vi "Preset_Manager_Main.vi"(4 "Virtual Devices List":string[](array[string]), 6 "Filtered Devices List":string[](array[string]), 8 "Experiment Name":string, 10 "DevStatusQueue":refnum<queue>, 11 "Software Root":string) -> ()   [LabVIEW 2020]
uses:
  <vilib>/Utility/miscctls.llb/LVRowAndColumnTypeDef.ctl
  Preset Query Enum.ctl
  <vilib>/Platform/browser.llb/Open URL in Default Browser (string).vi
  <userlib>/_OpenG.lib/array/array.llb/Delete Elements from 1D Array (String)__ogtk.vi
  <userlib>/_OpenG.lib/array/array.llb/Empty 1D Array (String)__ogtk.vi
panel:
  out "Queue Progress Bar":ext(slide) scale=0.0..1.0
  out "Queue Size":i32
  out "Current Preset Queue Element":string
  in  "Expt Devices Not On":i32(listbox)
  in  "Preset Devices Not in Experiment":i32(listbox)
  out "Active Preset":string
  out "Preset Execution Indicator":bool
  in  "EXIT":bool
  in  "Using Queue":bool
  in  "Tab Control":T1(tab)
  in  "Execute Preset":bool
  in  "Delete Preset":bool
  in  "Save as Preset":bool
  in  "Preset Menu":u16(ring) items=["None", "Pulsed Alignment", "3J", "Diode", "26J", "SingleShot", "1Hz", "800 MAX ND", "Amp3-8J-CapExit", "SDI", "CapInHexPosition", "CapOutHexFiberPosition", "Full Heater, Frog Out", "Full Heater, Frog In", "MagSpecSimulateBoff", "Pulsed", "CW", "Amp2, Clunker In", "Amp3-17J", "MagSpecSimulateBon", "SMFiber-In", "SMFiber-Out", "Amp3-MegaAttenuator", "developer", "developer_main", "developer_test_1", "dev_simcam_2", "dev_simcam_3"]
  in  "Load ECS to Table":bool
  in  "Navigate to ECS File":path
  in  "Preset Table Control":string[][](table)
  in  "Choose Values":bool
  in  "Left Join":bool
  in  "Reset Queue":bool
  in  "Queue Table Control":string[][](table)
  in  "Queue Table":string[][](table)
  in  "Execute Queue":bool
  in  "HELP WEB PAGE":bool
  out "PRESET FROM DB":string[][](table)
  out "ECS File":string[][](table)
  out "Coordinate Array":i32[][](array[numeric])
  out "Devices not started":string[](array[string]) caption="Devices not ready for scan"
  out "Active Device array":bool[](array[boolean])
  out "Active Dev/IP":string[](array[string])
  out "Device Errors":string[][](array[string])
  out "Queue Element":i32
  in  "Poll Count":i32
  in  "Mcast address":string
  in  "MCast Remote":u16
  in  "UDP timeout ms":i32
  in  "MC Multicast":refnum<k16>
  in  "My IP":string
  in  "All Devices Core Info":string[][](array[string])
  out "error out":errorcluster
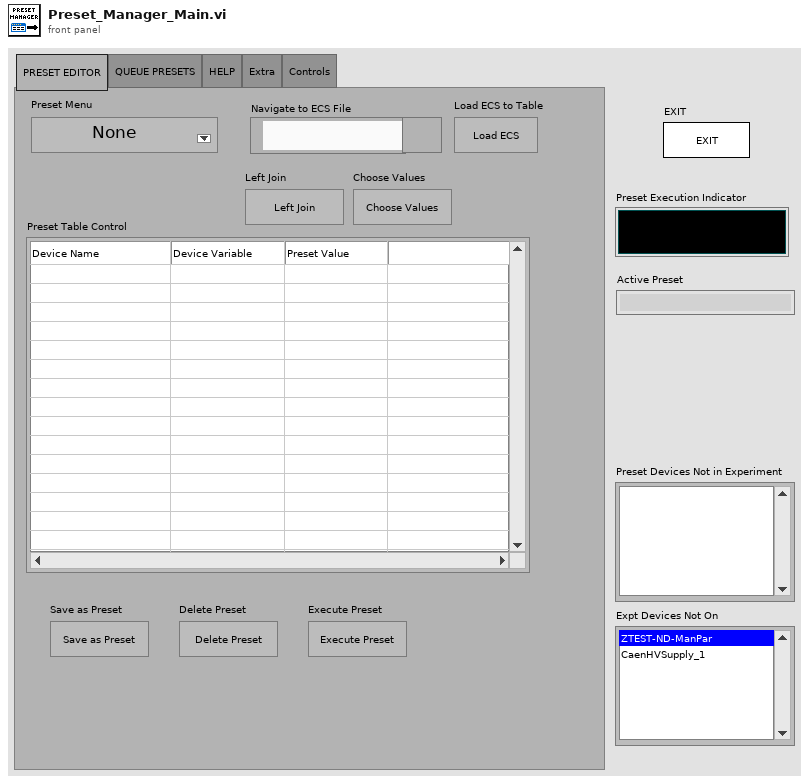
[diagram p1: front panel]
types:
  T1 = enum32{"PRESET EDITOR", "QUEUE PRESETS", "HELP", "Extra", "Controls"}
  T2 = typedef "LVRowAndColumnTypeDef.ctl" = cluster{"Row":i32, "Column":i32}
  T3 = typedef "Preset Query Enum.ctl" = enum16{"Get Locations", "Get all IPs and MACs", "Get classes", "Get expt variables to set at scanstart for particular device", "Get expt devices and variables with start values", "Get expt devices and variables (with data to get)", "Get expt devices with data to get", "Get Expt devices and GUIs", "Get all devices basic properties", "Get Virtual Devices Core Info", "Get Expt names", "Get experiment basic properties", "Get experiment alarm variables", "Get MC Ports", "Get device network comm port", "Get devicetype lvclass path", "Get basic device properties", "Get Init Order", "Get all setable variables of a device", "Get device variable aliases", "Get force values of all settable variables", "Get all variables of a devicetype", "Get all variables of a device", "Get plotter details", "Get Saved Scans", "Get Scan Info", "GetGeneralGUIs", "Get expt for plotter", "Get plotter IDs from expt", "Get all devices", "Get all Virtual Devices", "Get all aliases", "Get variable and device info for Virtual Device", "GetItemLocatorIP", "Get IPs for GUIs", "Get DeviceType from Device", "GetLocalPortRange", "GetDevicePresetVariables", "Get Device Configuration", "GetAllPresetNames", "GetAllConfigurationNames", "GetPresetDeviceNames", "GetDeviceAliases", "GetDevicesOfClass"}
  T4 = enum32{"Invalid", "Standard", "Closed", "Hidden", "Minimized", "Maximized"}
  T5 = enum32{"invalid app kind", "Development System", "Run Time System", "Student Edition", "Embedded LabVIEW", "Evaluation", "Custom"}
  T6 = cluster{"Core":cluster{"Current VI Reference":refnum<vi>, "Close Panel on Exit?":bool}, "Your Boolean data":bool, "String":string, "Preset Table Control":string[][], "Column Headers[]":string[], "Queue Table Control":string[][], "Preset Manager Cluster":cluster{"PresetName":string, "Mcast command":string, "Current Preset Devices":string[], "My IP":string, "Mcast address":string, "Software Root":string, "Experiment Name":string, "MCast Remote":u16, "UDP timeout ms":i32, "MC Multicast":refnum<k16>, "All Devices Core Info":string[][], "Filtered Devices List":string[], "Virtual Devices List":string[], "DevStatusQueue":refnum<queue>}}
  T7 = typedef "LVPoint32TypeDef.ctl" = cluster{"Horizontal":i32, "Vertical":i32}
  T8 = cluster{"Current VI Reference":refnum<vi>, "Close Panel on Exit?":bool}
  T9 = cluster{"PresetName":string, "Mcast command":string, "Current Preset Devices":string[], "My IP":string, "Mcast address":string, "Software Root":string, "Experiment Name":string, "MCast Remote":u16, "UDP timeout ms":i32, "MC Multicast":refnum<k16>, "All Devices Core Info":string[][], "Filtered Devices List":string[], "Virtual Devices List":string[], "DevStatusQueue":refnum<queue>}
  T10 = enum16{"Left Button", "Center Button", "Right Button", "Window Close"}
  T11 = typedef "mysql_authentication.ctl" = cluster{"User":string, "Password":string, "Database":string}
  T12 = cluster{"Port":u16, "IP Address":string, "Authentication":T11}
  T13 = typedef "preset diagnostics.ctl" = cluster{"Active Preset Achieved":bool, "Devices with Active Preset Not Set":string[], "Dev Presets":string[], "All Preset Devices ON?":bool[]}
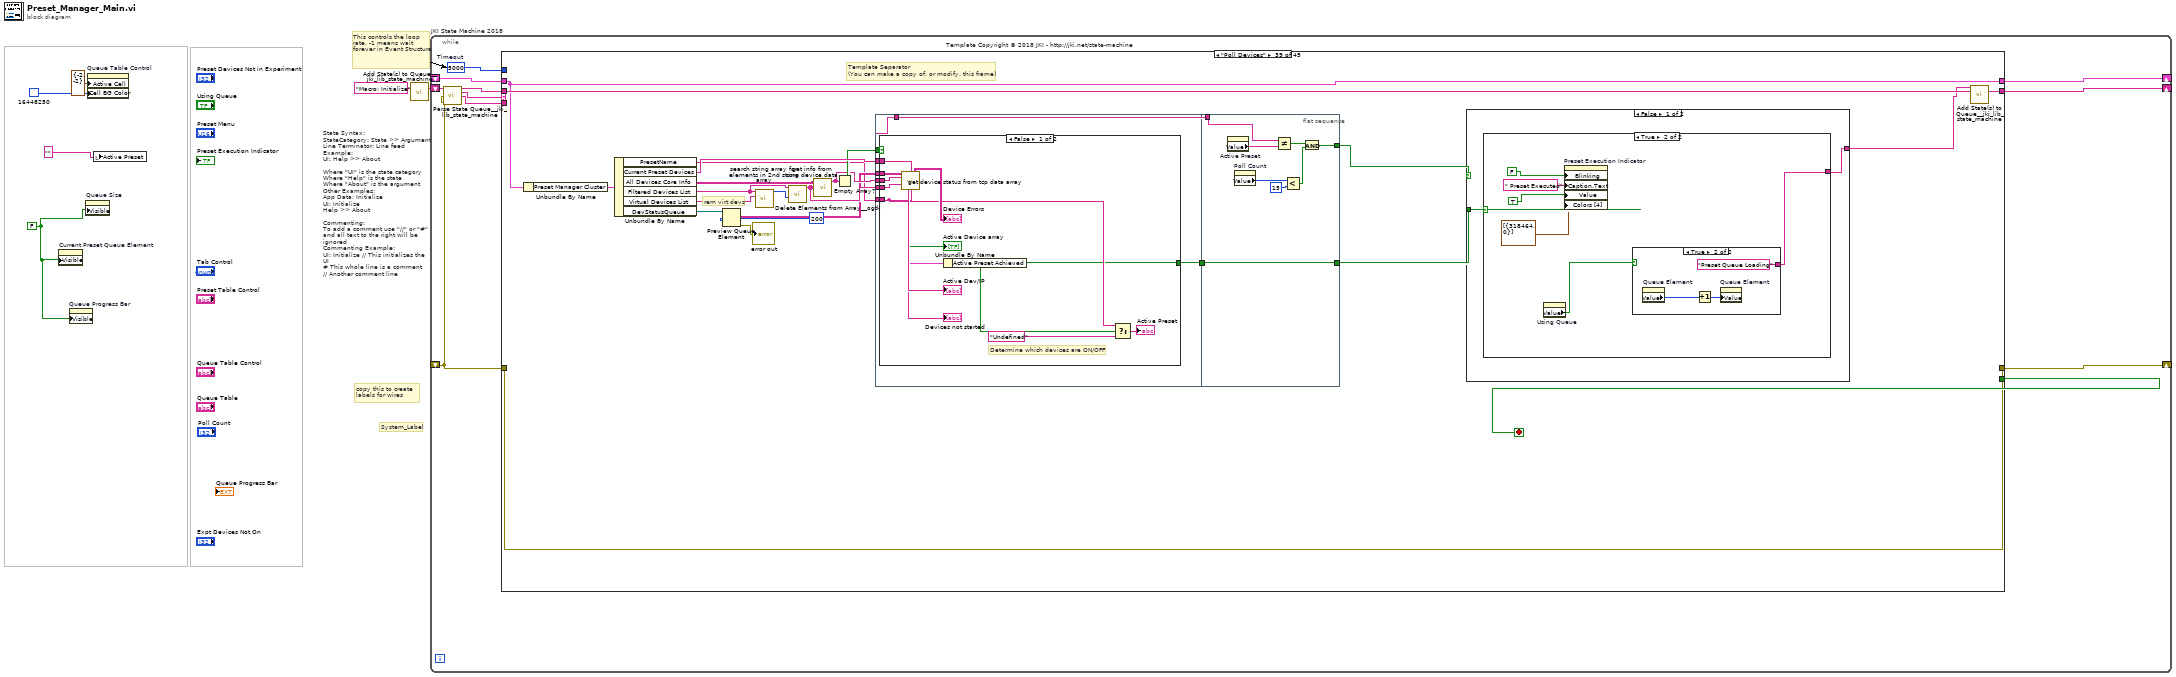
[diagram p0: block diagram]
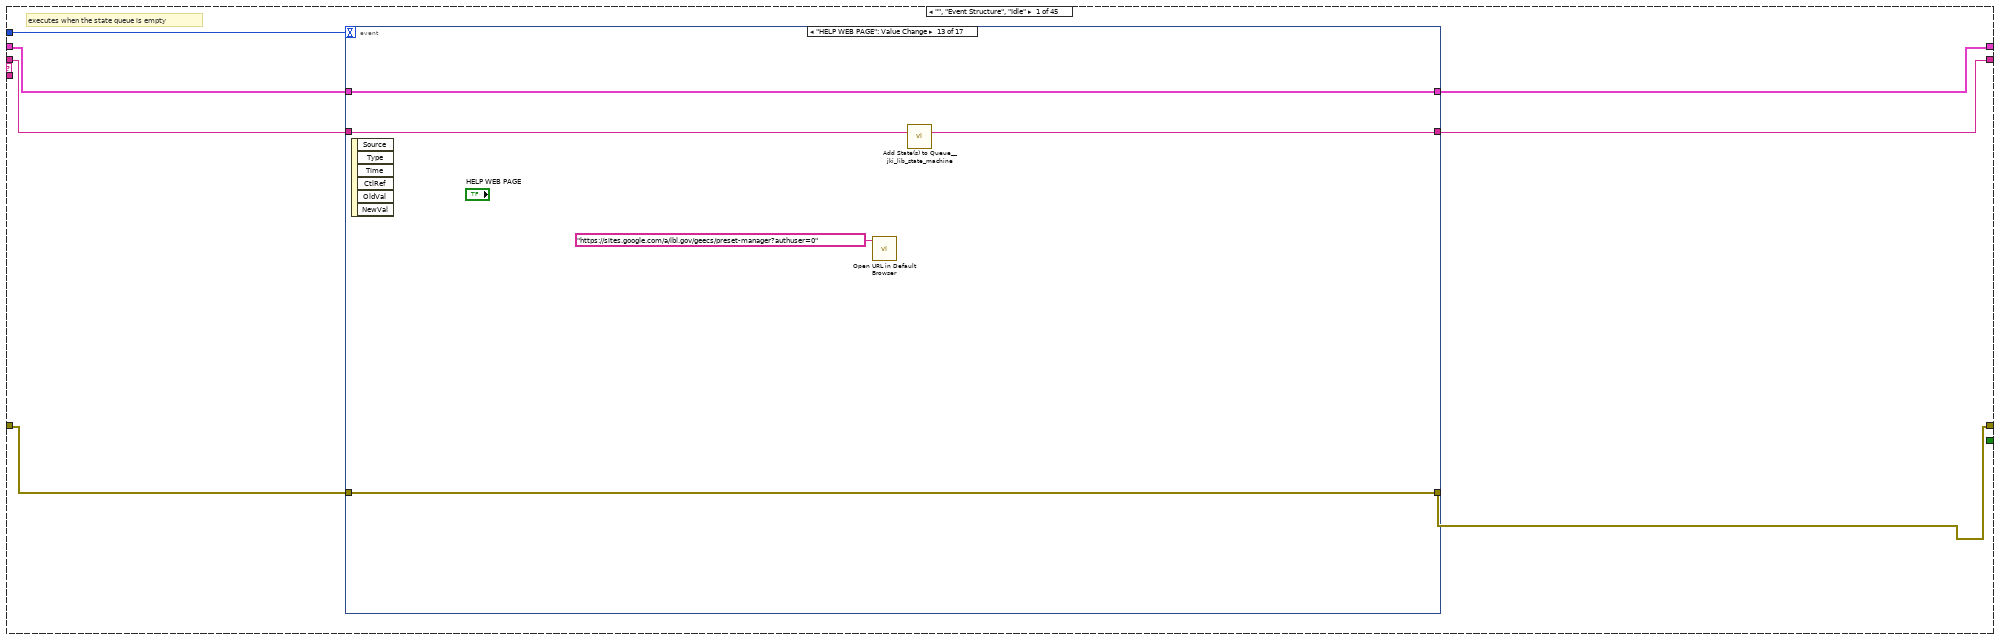
[diagram p2: hidden frame]
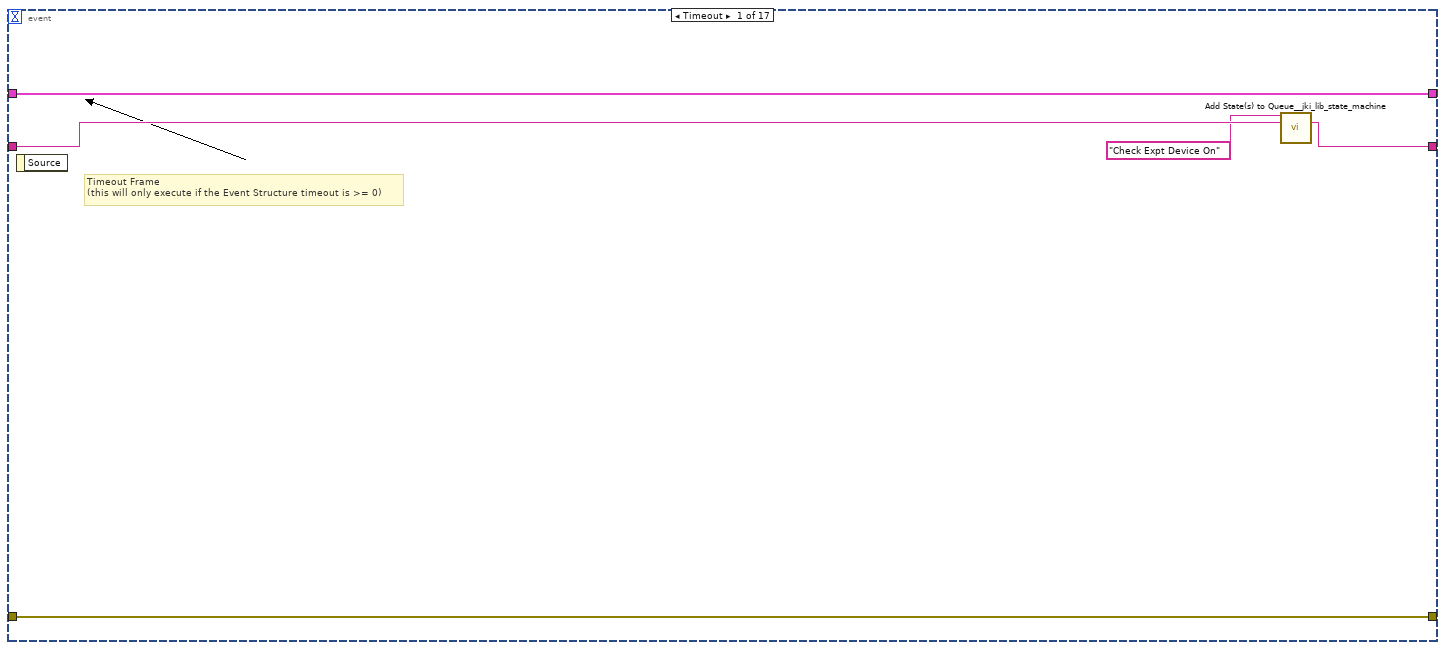
[diagram p3: hidden frame]
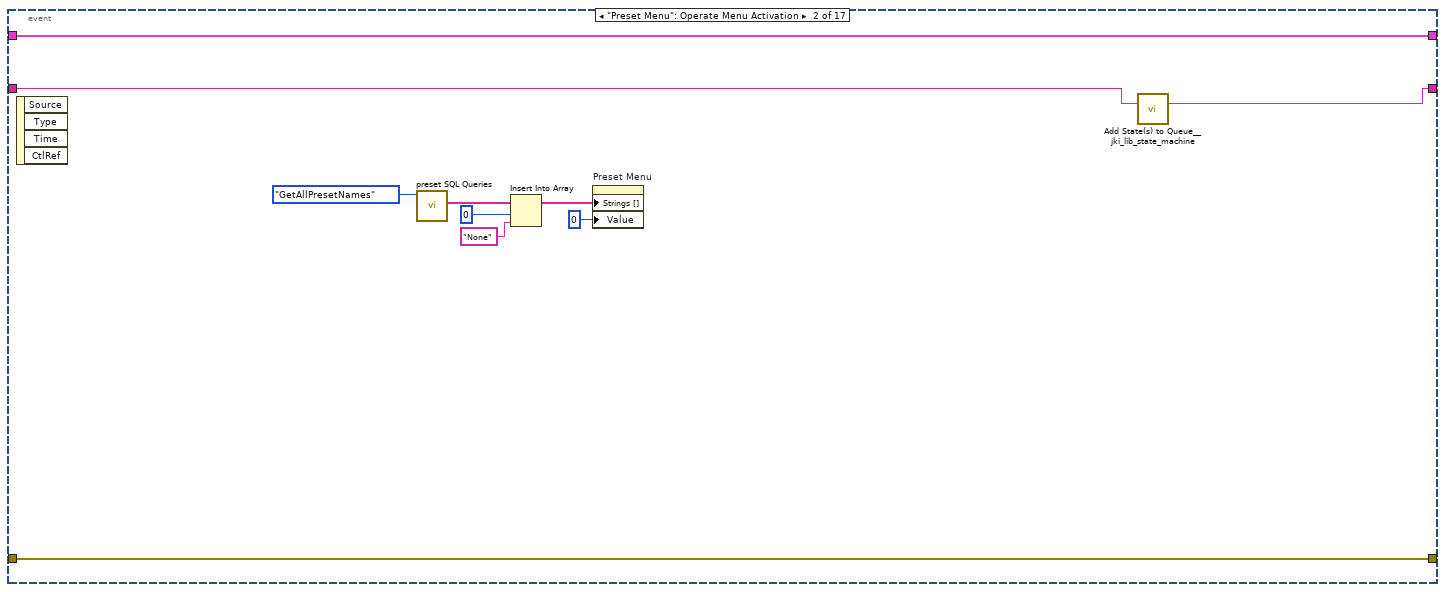
[diagram p4: hidden frame]
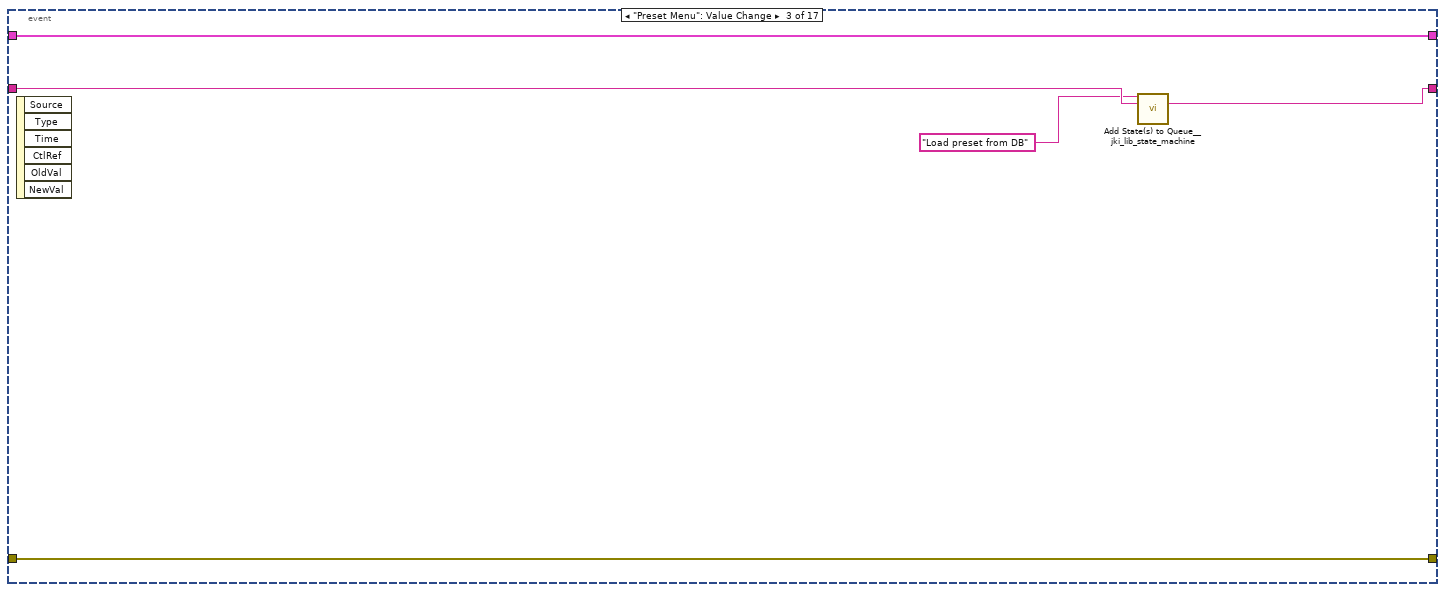
[diagram p5: hidden frame]
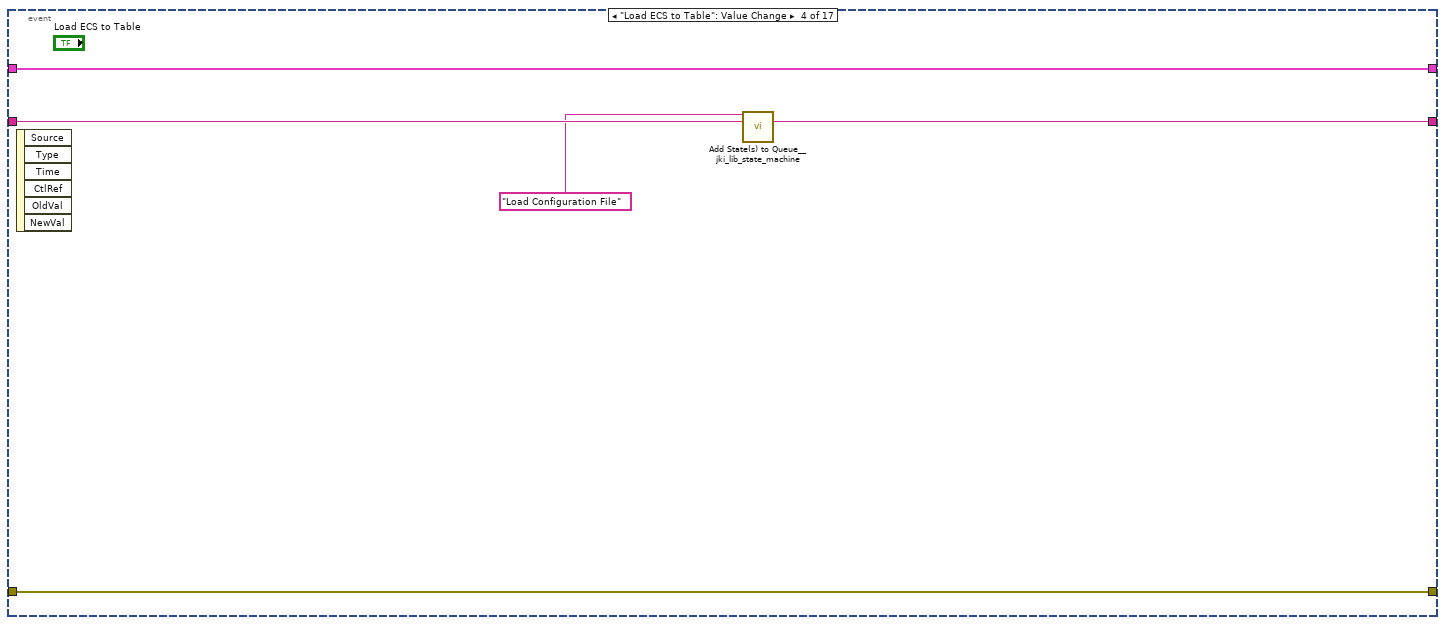
[diagram p6: hidden frame]
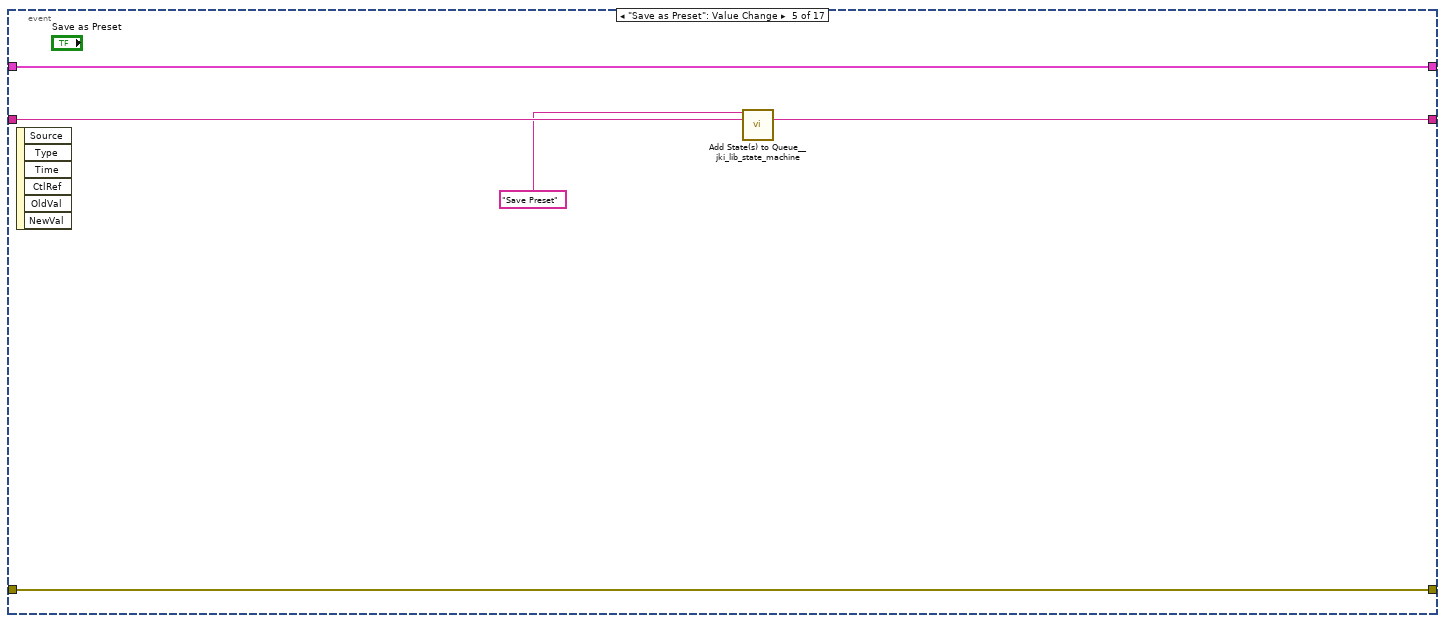
[diagram p7: hidden frame]
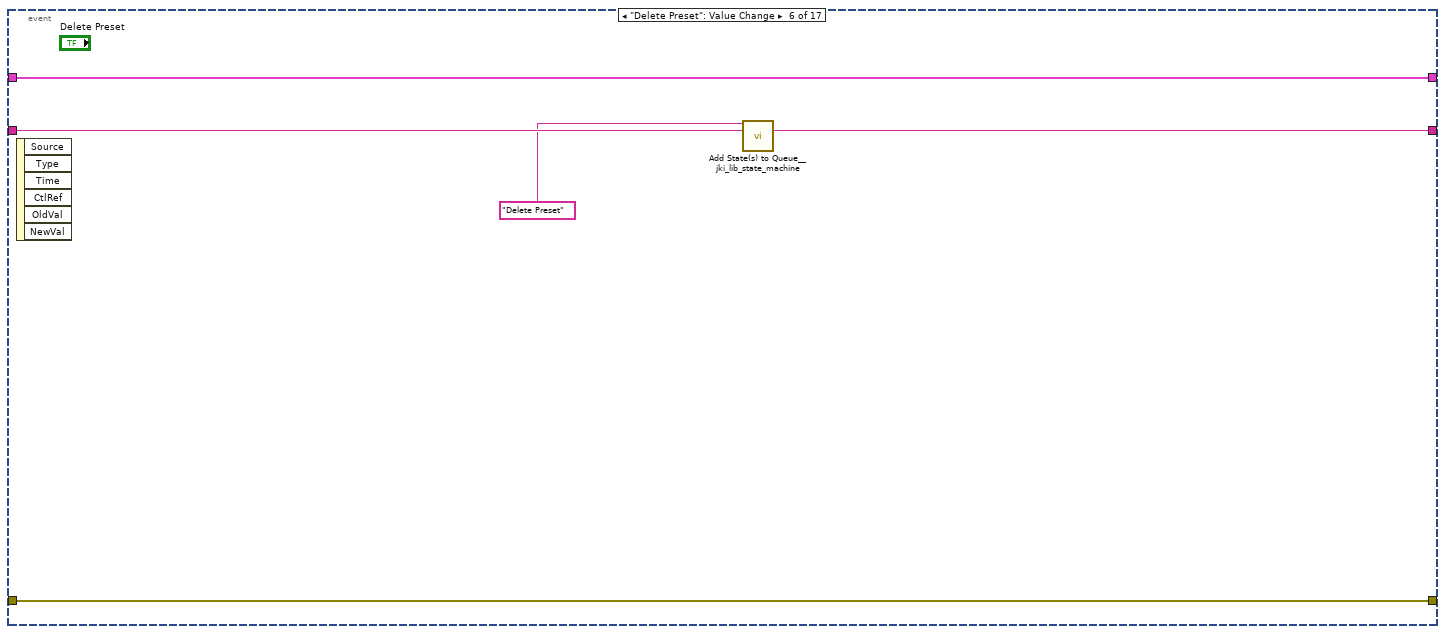
[diagram p8: hidden frame]
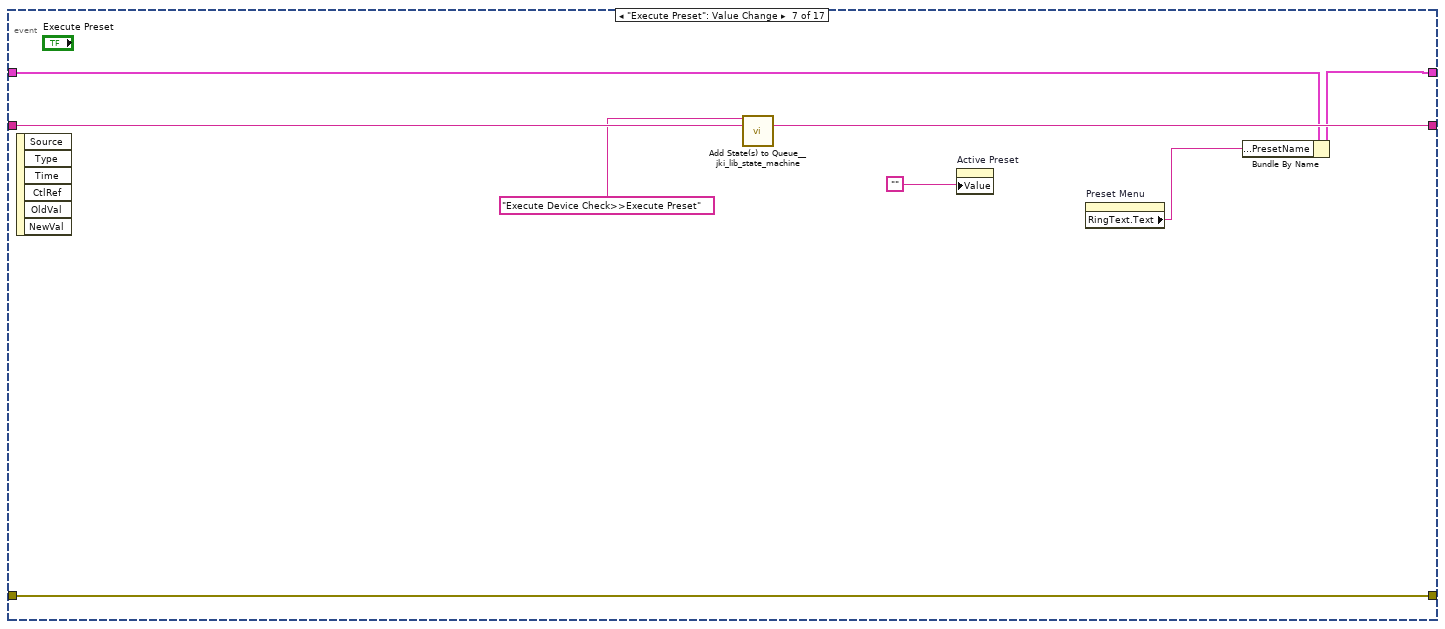
[diagram p9: hidden frame]
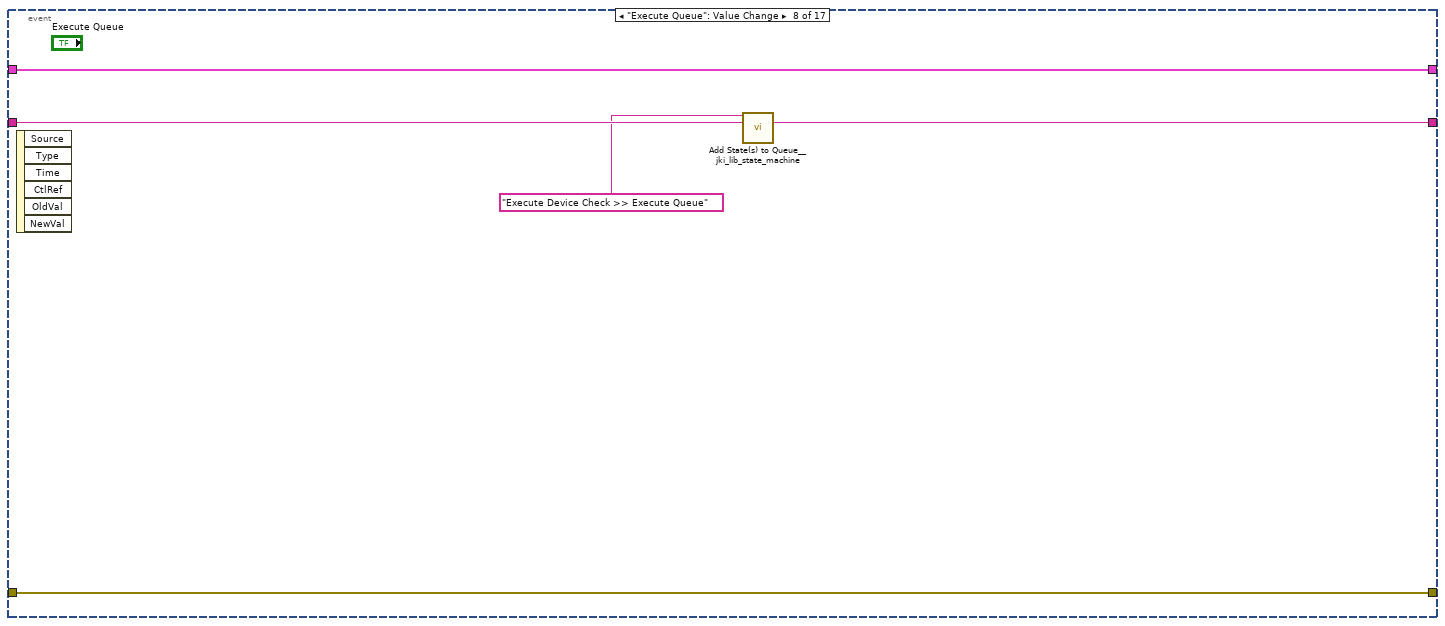
[diagram p10: hidden frame]
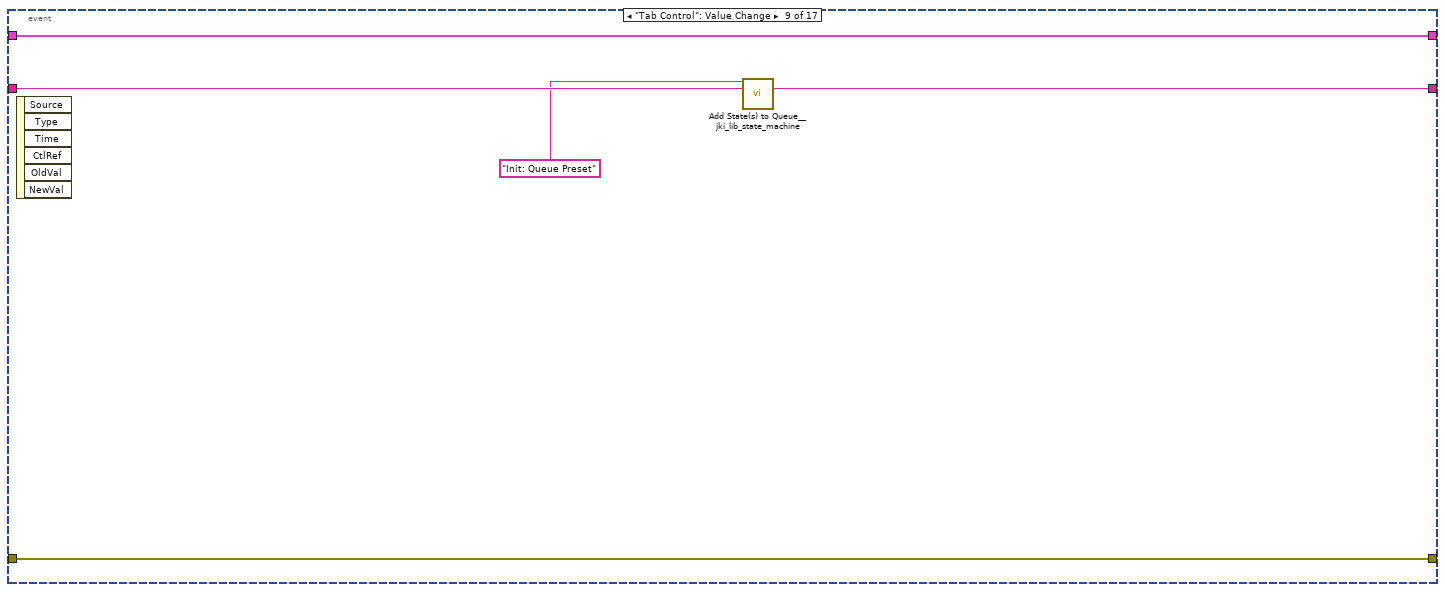
[diagram p11: hidden frame]
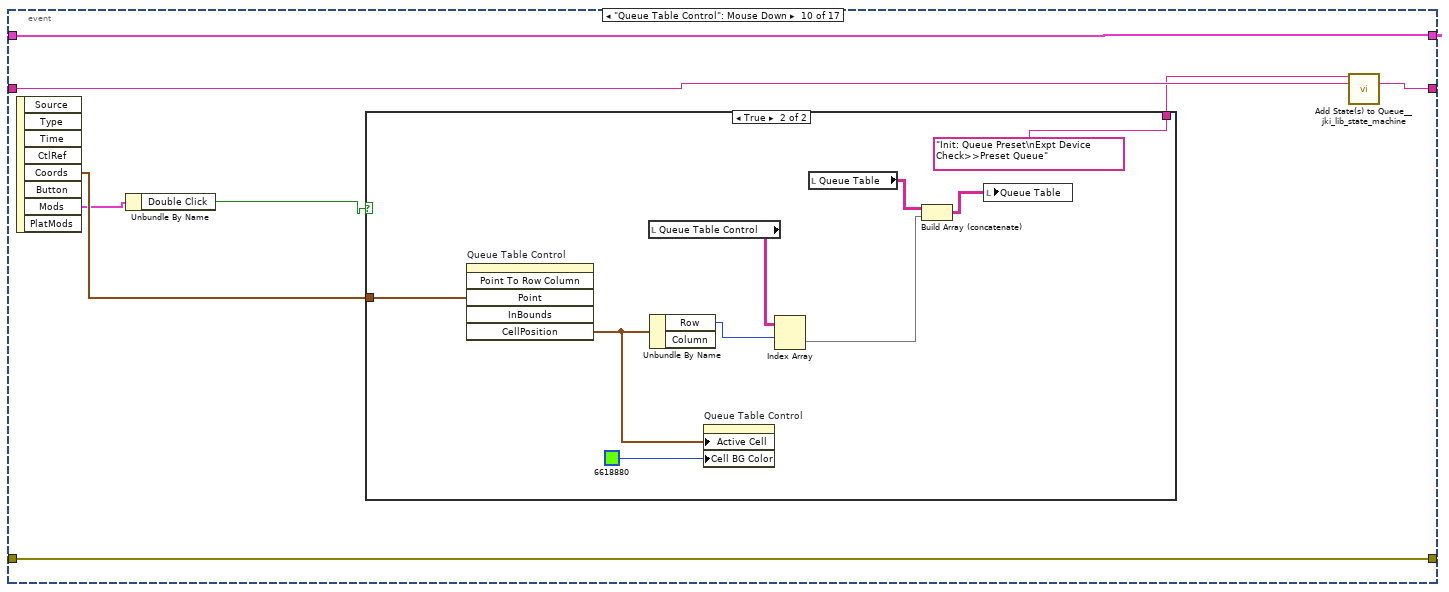
[diagram p12: hidden frame]
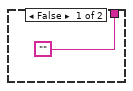
[diagram p13: hidden frame]
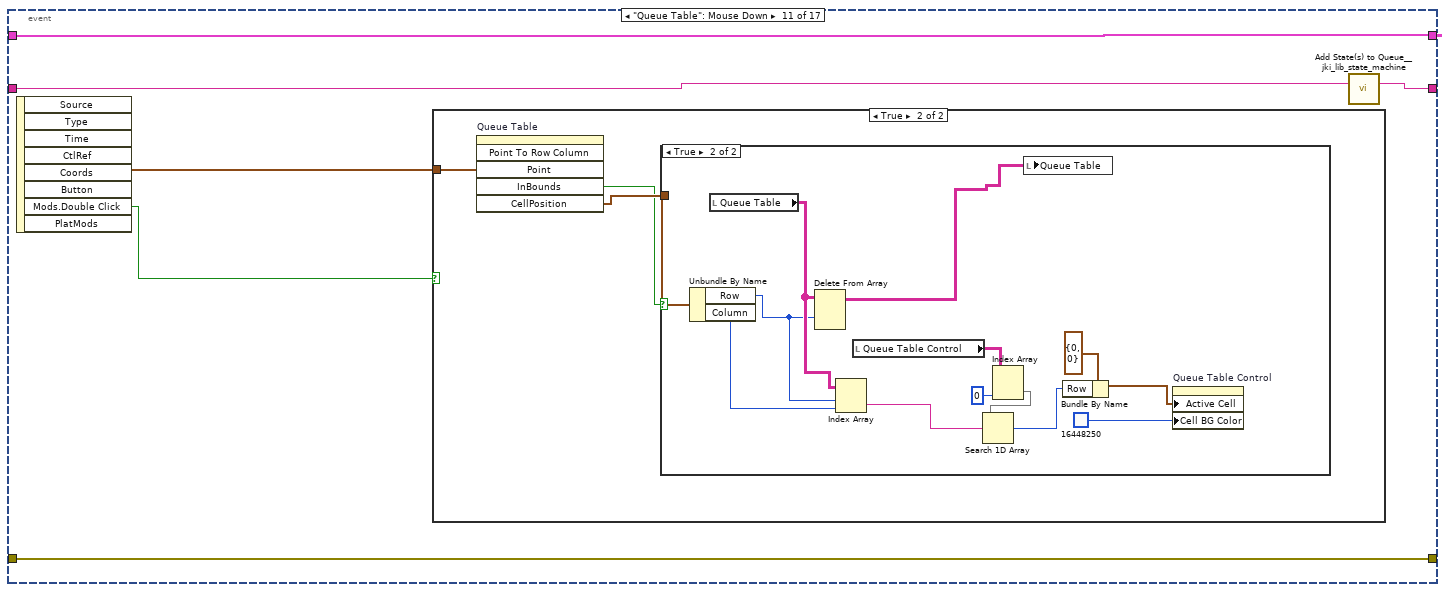
[diagram p14: hidden frame]
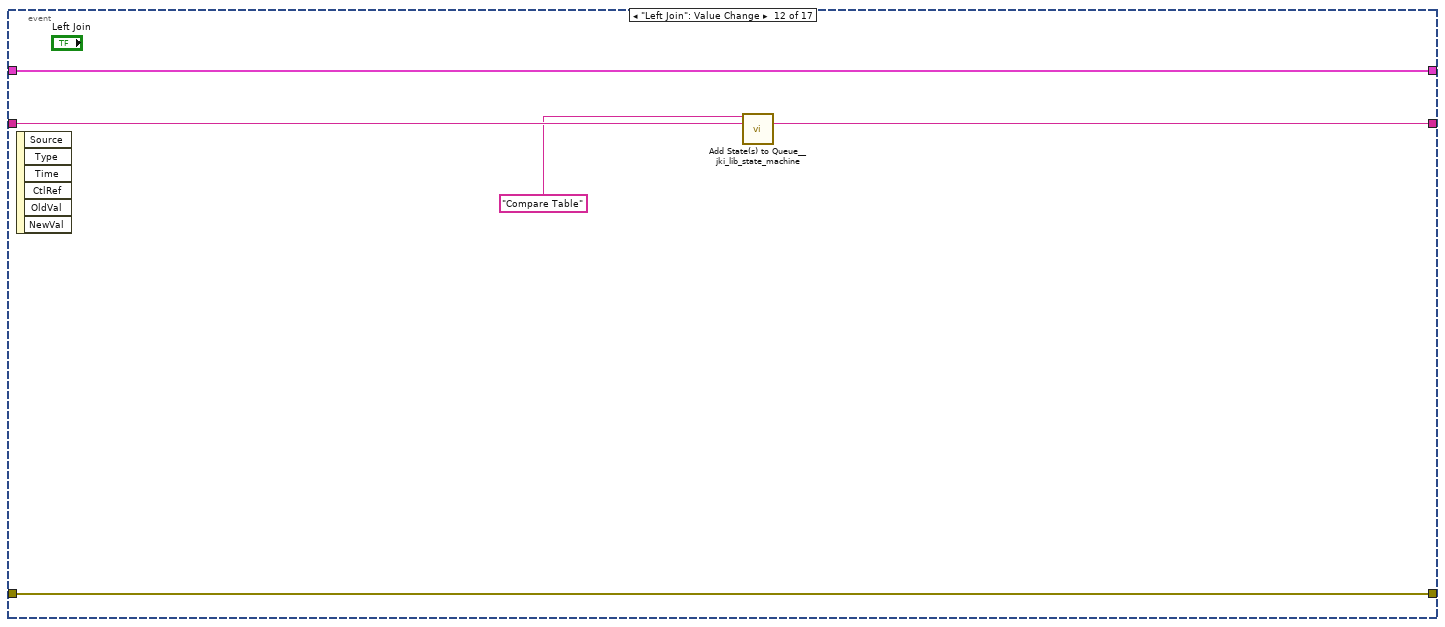
[diagram p17: hidden frame]
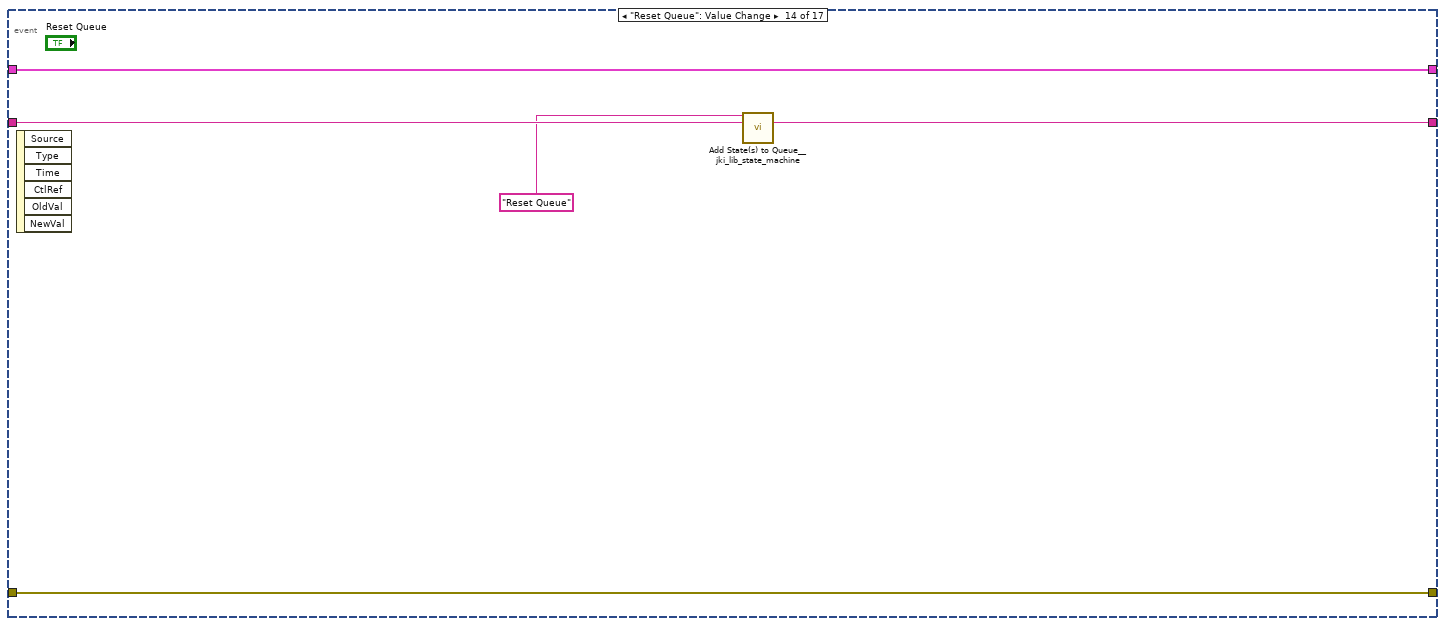
[diagram p18: hidden frame]
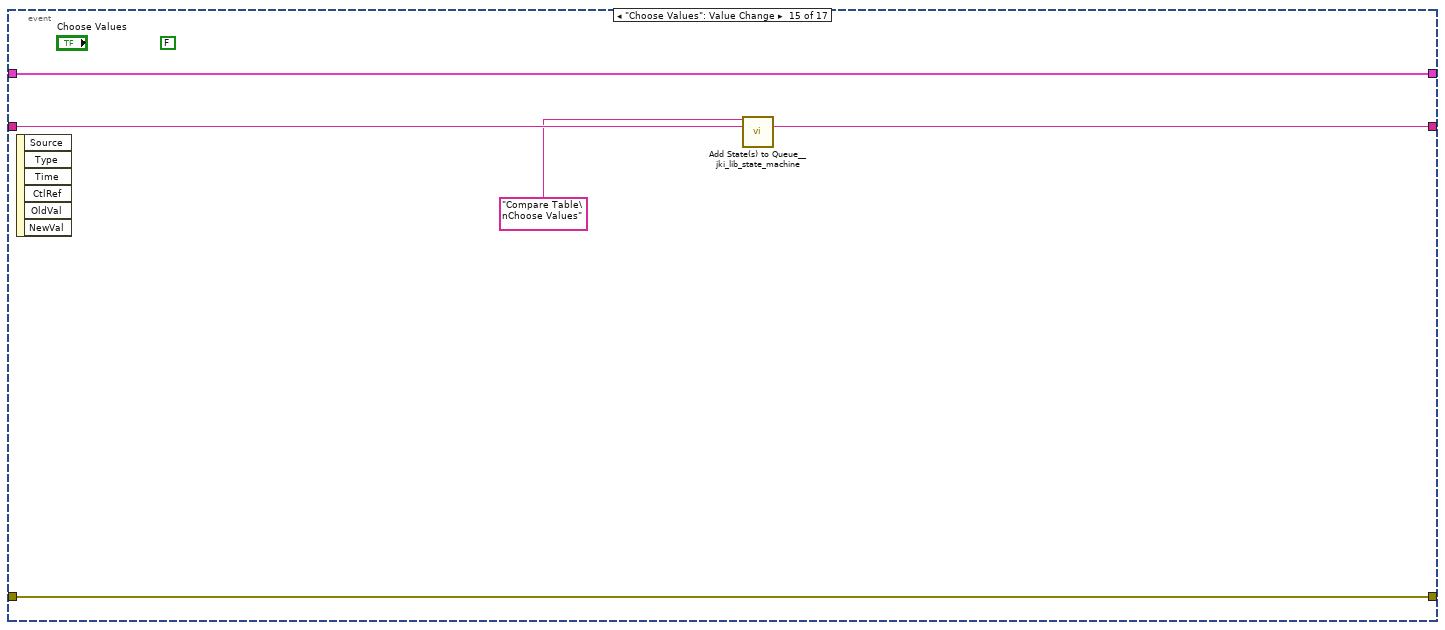
[diagram p19: hidden frame]
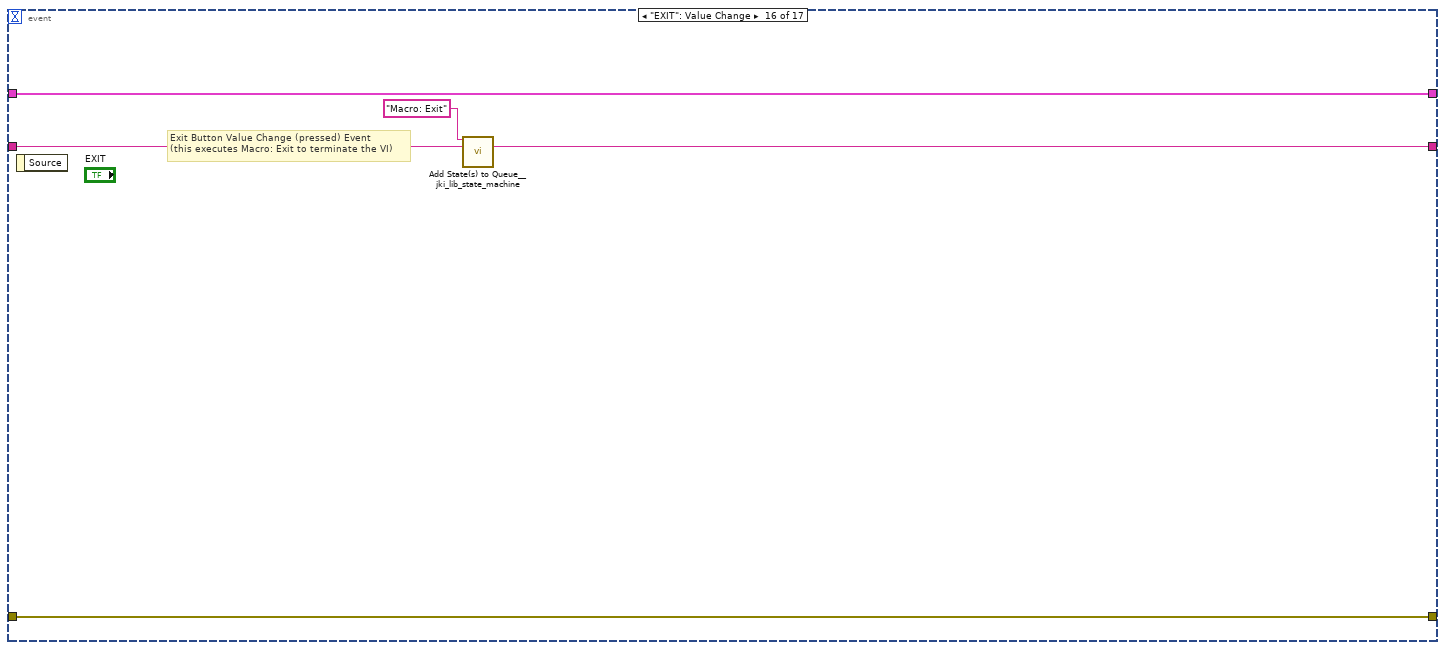
[diagram p20: hidden frame]
diagram:
  w1 = FALSE
  # "State Syntax:\nStateCategory: State >> Argument\nLine Terminator: Line feed\nExample:\nUI: Help >> About\n\nWhere \"UI\" is the state category\nWhere \"Help\" is the state\nWhere \"About\" is the argument\nOther Examples:\nApp Data: Initialize\nUI: Initialize\nHelp >> About\n\nCommenting:\nTo add a comment use \"//\" or \"#\" and all text to the right will be ignored\nCommenting Example:\nUI: Initialize // This initializes the UI\n# This whole line is a comment\n// Another comment line"
  # "copy this to create labels for wires"
  # "This controls the loop rate. -1 means wait forever in Event Structure"
  # "System_Label"
  n1 = property on="Current Preset Queue Element" class="Str"("Visible"=w1) -> ()  [unwired: 2 in, 2 out]
  n2 = property on="Queue Progress Bar" class="Slide (strict)"("Visible"=w1) -> ()  [unwired: 2 in, 2 out]
  n3 = property on="Queue Size" class="DigNum (strict)"("Visible"=w1) -> ()  [unwired: 2 in, 2 out]
  n4 = property on="Queue Table Control" class="Tbl (strict)"("Active Cell"=T2 {"Row"=-2, "Column"=-2} ("Active Cell:Active Cell"), "Cell BG Color"=u32 16448250 ("Active Cell:Cell Background Color")) -> ()  [unwired: 2 in, 2 out]
  n5 = local write "Active Preset"("" ("My IP")) -> ()
  n6 = call <vilib>:"Add State(s) to Queue__jki_lib_state_machine.vi"("State(s) in (\"\")"="Macro: Initialize") -> ("States Out"=w6:string)  [unwired: 14 in]
  n7 = while "JKI State Machine 2018" {
    shift-right: [w7] -> _
    shift-left: _ -> [w10]
    shift-right: [w13] -> _
    shift-left: _ -> [w8]
    shift-right: [w12] -> _
    shift-left: w6 -> [w14]
    stop <- w11 stop-if-true
    w9 = 5000  # Timeout
    # "Template Copyright © 2018 JKI - http://jki.net/state-machine"
    n8 = call <vilib>:"Parse State Queue__jki_lib_state_machine.vi"("State Queue"=w14, "Error In (no error)"=w8) -> ("Remaining States"=w16:string, "Current State"=w17:string, "Arguments"=w15:string)  [unwired: 11 in]
    n9 = case shown="\"Poll Devices\"" w17 {
      selector: w17 -> [_ _ w153 _ _ _ _ _ _ _ _ _ _ _ _ _ _ _ _ _ _ _ _ _ _ _ _ _ _ _ _ _ _ _ _ _ _ _ _ _ _ _ _ _ _]
      tunnel: w16 -> [w24 w152 w157 w176 w182 w187 w191 w208 w214 w218 w222 w228 w239 w308 w319 w329 w341 w345 w355 w363 w373 w382 w391 w401 w418 w444 w478 w493 w497 w503 w507 w514 w523 w528 w543 w570 w575 w591 w614 w677 w689 w693 w699 w724 w757]
      tunnel: w15 -> [_ _ _ _ _ _ _ _ _ _ _ w223 w233 _ _ _ _ _ _ _ _ _ _ _ _ _ _ _ _ _ _ _ _ _ _ _ _ w585 _ _ _ _ w695 w720 _]
      tunnel: w10 -> [w22 w149 w155 w169 w179 w185 w188 _ w209 w215 w220 w226 w235 w305 w316 w326 w338 w342 w350 w356 w369 w379 w387 w398 w415 w441 w474 w490 w494 w500 w504 w509 w520 w525 w539 w567 w572 w588 w610 w670 w680 w690 w696 w721 w754]
      tunnel: [w21 w150 w159 w173 errorcluster {"status"=FALSE, "code"=0, "source"=""} ("error out") w184 w189 w206 w210 w216 w219 w224 w236 w306 w317 w327 w339 w343 w353 w361 w371 w380 w389 w399 w416 w442 w476 w491 w495 w501 w505 w512 w521 w526 w541 w568 w573 w589 w612 w675 w687 w691 w697 w722 w755] -> w13
      tunnel: w8 -> [w20 w150 w158 w173 w178 w184 w189 w206 w211 w216 w219 w225 w237 w306 w317 w327 w339 w343 w353 w361 w371 w380 w389 w399 w416 w442 w476 w491 w495 w501 w505 w512 w521 w526 w541 w568 w573 w589 w612 w675 w687 w691 w697 w722 w755]
      tunnel: [w23 w151 w156 w175 w181 w186 w190 w207 w213 w217 w221 w227 w238 w307 w318 w328 w340 w344 w354 w362 w372 w381 w390 w400 w417 w443 w477 w492 w496 w502 w506 w513 w522 w527 w542 w569 w574 w590 w613 w676 w688 w692 w698 w723 w756] -> w12
      tunnel: [_ _ _ _ _ TRUE _ _ _ _ _ _ _ _ _ _ _ _ _ _ _ _ _ _ _ _ _ _ _ _ _ _ _ _ _ _ _ _ _ _ _ _ _ _ _] -> w11
      tunnel: w9 -> [w18 _ _ _ _ _ _ _ _ _ _ _ _ _ _ _ _ _ _ _ _ _ _ _ _ _ _ _ _ _ _ _ _ _ _ _ _ _ _ _ _ _ _ _ _]
      tunnel: [w19 w149 w155 w174 w179 w185 w188 w197 w209 w215 w220 w226 w235 w305 w316 w326 w337 w342 w348 w356 w368 w378 w386 w398 w415 w441 w474 w490 w494 w500 w504 w509 w520 w525 w538 w567 w571 w588 w610 w671 w679 w690 w696 w721 w754] -> w7
      frame "", "Event Structure", "Idle" {
        # "executes when the state queue is empty"
        n10 = event shown="[12] \"HELP WEB PAGE\": Value Change" {
          selector: _ -> [_ _ _ _ _ _ _ _ _ _ _ _ _ _ _ _ _]
          dyn-events: _ -> [_ _ _ _ _ _ _ _ _ _ _ _ _ _ _ _ _]
          timeout: w18 -> [_ _ _ _ _ _ _ _ _ _ _ _ _ _ _ _ _]
          tunnel: w24 -> [w29 w31 w42 w47 w52 w57 w66 w70 w76 w84 w100 w120 w125 w130 w135 w142 w148]
          tunnel: [w28 w30 w41 w46 w51 w56 w65 w69 w75 w83 w99 w119 w124 w129 w134 w141 w147] -> w23
          tunnel: w22 -> [w26 w39 w44 w49 w54 w59 w61 w72 w73 w81 w98 w122 w127 w132 w137 w139 w145]
          tunnel: [w27 w38 w43 w48 w53 w58 w67 w71 w77 w85 w101 w121 w126 w131 w136 w140 w146] -> w21
          tunnel: w20 -> [w27 w38 w43 w48 w53 w58 w67 w71 w77 w85 w101 w121 w126 w131 w136 w140 w146]
          tunnel: [w26 w39 w44 w49 w54 w59 w60 w72 w73 w81 w98 w122 w127 w132 w137 w139 w145] -> w19
          event Timeout {
            # "Timeout Frame\n(this will only execute if the Event Structure timeout is >= 0)"
            n11 = event-data() -> ()  [unwired: 1 in, 1 out]
            n12 = call <vilib>:"Add State(s) to Queue__jki_lib_state_machine.vi"("State(s) in Front (\"\")"="Check Expt Device On" ("State(s) in Front (\"\")"), "State(s) in (\"\")"=w29) -> ("States Out"=w28:string)  [unwired: 13 in]
          }
          event "Preset Menu": Operate Menu Activation {
            n13 = event-data() -> ()  [unwired: 1 in, 4 out]
            n14 = call "preset SQL Queries.vi"("Preset Query"=Preset_Query_Enum."GetAllPresetNames") -> ("1st column 1st data"=w36:string[])  [unwired: 8 in, 2 out]
            n15 = Insert Into Array(array=w36, index=0, new element="None" ("new element/subarray")) -> (w33:string[])
            n16 = property on="Preset Menu" class="Ring (strict)"("Strings []"=w33, "Value"=0 ("index")) -> ()  [unwired: 2 in, 2 out]
            n17 = call <vilib>:"Add State(s) to Queue__jki_lib_state_machine.vi"("State(s) in (\"\")"=w31) -> ("States Out"=w30:string)  [unwired: 14 in]
          }
          event "Preset Menu": Value Change {
            n18 = event-data() -> ()  [unwired: 1 in, 6 out]
            n19 = call <vilib>:"Add State(s) to Queue__jki_lib_state_machine.vi"("State(s) in Front (\"\")"="Load preset from DB" ("State(s) in Front (\"\")"), "State(s) in (\"\")"=w42) -> ("States Out"=w41:string)  [unwired: 13 in]
          }
          event "Load ECS to Table": Value Change {
            n20 = event-data() -> ()  [unwired: 1 in, 6 out]
            n21 = call <vilib>:"Add State(s) to Queue__jki_lib_state_machine.vi"("State(s) in Front (\"\")"="Load Configuration File", "State(s) in (\"\")"=w47) -> ("States Out"=w46:string)  [unwired: 13 in]
          }
          event "Save as Preset": Value Change {
            n22 = event-data() -> ()  [unwired: 1 in, 6 out]
            n23 = call <vilib>:"Add State(s) to Queue__jki_lib_state_machine.vi"("State(s) in Front (\"\")"="Save Preset", "State(s) in (\"\")"=w52) -> ("States Out"=w51:string)  [unwired: 13 in]
          }
          event "Delete Preset": Value Change {
            n24 = event-data() -> ()  [unwired: 1 in, 6 out]
            n25 = call <vilib>:"Add State(s) to Queue__jki_lib_state_machine.vi"("State(s) in Front (\"\")"="Delete Preset", "State(s) in (\"\")"=w57) -> ("States Out"=w56:string)  [unwired: 13 in]
          }
          event "Execute Preset": Value Change {
            n26 = event-data() -> ()  [unwired: 1 in, 6 out]
            n27 = call <vilib>:"Add State(s) to Queue__jki_lib_state_machine.vi"("State(s) in Front (\"\")"="Execute Device Check>>Execute Preset", "State(s) in (\"\")"=w66) -> ("States Out"=w65:string)  [unwired: 13 in]
            n28 = property on="Active Preset" class="Str"("Value"="") -> ()  [unwired: 2 in, 2 out]
            n29 = property on="Preset Menu" class="Ring (strict)"() -> ("RingText.Text"=w62:string)  [unwired: 2 in, 2 out]
            n30 = Bundle By Name(cluster=w61, "Preset Manager Cluster.PresetName"=w62) -> (w60:T6)
          }
          event "Execute Queue": Value Change {
            n31 = event-data() -> ()  [unwired: 1 in, 6 out]
            n32 = call <vilib>:"Add State(s) to Queue__jki_lib_state_machine.vi"("State(s) in Front (\"\")"="Execute Device Check >> Execute Queue", "State(s) in (\"\")"=w70) -> ("States Out"=w69:string)  [unwired: 13 in]
          }
          event "Tab Control": Value Change {
            n33 = event-data() -> ()  [unwired: 1 in, 6 out]
            n34 = call <vilib>:"Add State(s) to Queue__jki_lib_state_machine.vi"("State(s) in Front (\"\")"="Init: Queue Preset", "State(s) in (\"\")"=w76) -> ("States Out"=w75:string)  [unwired: 13 in]
          }
          event "Queue Table Control": Mouse Down {
            n35 = event-data() -> ("Coords"=w80:T7, "Mods"=w79:cluster{"Double Click":bool, "Menu Key":bool})  [unwired: 1 in, 6 out]
            n36 = Unbundle By Name(w79) -> ("Double Click"=w78:bool)
            n37 = case shown="True" w78 {
              tunnel: ["" "Init: Queue Preset\nExpt Device Check>>Preset Queue"] -> w82
              tunnel: w80 -> [_ w94]
              frame False {
              }
              frame True {
                n38 = invoke on="Queue Table Control" class="Tbl (strict)" method="Point To Row Column"("Point"=w94) -> ("CellPosition"=w91:T2)  [unwired: 5 in, 5 out]
                n39 = local read "Queue Table Control"() -> (w93:string[][])
                n40 = Unbundle By Name(w91) -> ("Row"=w92:i32)  [unwired: 1 out]
                n41 = property on="Queue Table Control" class="Tbl (strict)"("Active Cell"=w91, "Cell BG Color"=u32 6618880 ("Active Cell:Cell Background Color")) -> ()  [unwired: 2 in, 2 out]
                n42 = Index Array(array=w93, index (row)=w92) -> (element=w89:string[])  [unwired: 1 in]
                n43 = local read "Queue Table"() -> (w87:string[][])
                n44 = Build Array (concatenate)(w87, w89) -> (w88:string[][])
                n45 = local write "Queue Table"(w88) -> ()
              }
            }
            n46 = call <vilib>:"Add State(s) to Queue__jki_lib_state_machine.vi"("State(s) in Front (\"\")"=w82, "State(s) in (\"\")"=w84) -> ("States Out"=w83:string)  [unwired: 13 in]
          }
          event "Queue Table": Mouse Down {
            n47 = event-data() -> ("Coords"=w97:T7, "Mods.Double Click"=w96:bool)  [unwired: 1 in, 6 out]
            n48 = case shown="True" w96 {
              tunnel: w97 -> [_ w104]
              frame False {
              }
              frame True {
                n49 = invoke on="Queue Table" class="Tbl (strict)" method="Point To Row Column"("Point"=w104) -> ("InBounds"=w102:bool, "CellPosition"=w103:T2)  [unwired: 5 in, 4 out]
                n50 = case shown="True" w102 {
                  tunnel: w103 -> [_ w117]
                  frame False {
                  }
                  frame True {
                    n51 = Unbundle By Name(w117) -> ("Row"=w114:i32, "Column"=w113:i32)
                    n52 = local read "Queue Table"() -> (w115:string[][])
                    n53 = Delete From Array(array=w115, index (row)=w114) -> (array with subset deleted=w116:string[][])  [unwired: 2 in, 1 out]
                    n54 = Index Array(array=w115, index (row)=w114, index (col)=w113) -> (element=w112:string)
                    n55 = local read "Queue Table Control"() -> (w111:string[][])
                    n56 = Index Array(array=w111, index (col)=0 ("disabled index (col)")) -> (element=w109:string[])  [unwired: 1 in]
                    n57 = Search 1D Array(1D array=w109, element=w112) -> (index of element=w105:i32)  [unwired: 1 in]
                    n58 = local write "Queue Table"(w116) -> ()
                    n59 = Bundle By Name(cluster=T2 {"Row"=0, "Column"=0} ("Active Cell:Active Cell"), "Row"=w105) -> (w106:T2)
                    n60 = property on="Queue Table Control" class="Tbl (strict)"("Active Cell"=w106, "Cell BG Color"=u32 16448250 ("Active Cell:Cell Background Color")) -> ()  [unwired: 2 in, 2 out]
                  }
                }
              }
            }
            n61 = call <vilib>:"Add State(s) to Queue__jki_lib_state_machine.vi"("State(s) in (\"\")"=w100) -> ("States Out"=w99:string)  [unwired: 14 in]
          }
          event "Left Join": Value Change {
            n62 = event-data() -> ()  [unwired: 1 in, 6 out]
            n63 = call <vilib>:"Add State(s) to Queue__jki_lib_state_machine.vi"("State(s) in Front (\"\")"="Compare Table", "State(s) in (\"\")"=w120) -> ("States Out"=w119:string)  [unwired: 13 in]
          }
          event "HELP WEB PAGE": Value Change {
            n64 = event-data() -> ()  [unwired: 1 in, 6 out]
            n65 = call-poly <vilib>:"Open URL in Default Browser.vi"("URL"="https://sites.google.com/a/lbl.gov/geecs/preset-manager?authuser=0") -> ()  [unwired: 5 in, 2 out]
            n66 = call <vilib>:"Add State(s) to Queue__jki_lib_state_machine.vi"("State(s) in (\"\")"=w125) -> ("States Out"=w124:string)  [unwired: 14 in]
          }
          event "Reset Queue": Value Change {
            n67 = event-data() -> ()  [unwired: 1 in, 6 out]
            n68 = call <vilib>:"Add State(s) to Queue__jki_lib_state_machine.vi"("State(s) in Front (\"\")"="Reset Queue", "State(s) in (\"\")"=w130) -> ("States Out"=w129:string)  [unwired: 13 in]
          }
          event "Choose Values": Value Change {
            (unwired) FALSE ("Choose Values")
            n69 = event-data() -> ()  [unwired: 1 in, 6 out]
            n70 = call <vilib>:"Add State(s) to Queue__jki_lib_state_machine.vi"("State(s) in Front (\"\")"="Compare Table\nChoose Values", "State(s) in (\"\")"=w135) -> ("States Out"=w134:string)  [unwired: 13 in]
          }
          event "EXIT": Value Change {
            # "Exit Button Value Change (pressed) Event\n(this executes Macro: Exit to terminate the VI)"
            n71 = event-data() -> ()  [unwired: 1 in, 1 out]
            n72 = call <vilib>:"Add State(s) to Queue__jki_lib_state_machine.vi"("State(s) in Front (\"\")"="Macro: Exit", "State(s) in (\"\")"=w142) -> ("States Out"=w141:string)  [unwired: 13 in]
          }
          event Panel Close? {
            # "Discard the event because we'll close the front panel ourselves in Macro: Exit"
            # "Close Panel button (pressed) Event\n(this executes Macro: Exit to terminate the VI)"
            n73 = event-data() -> ()  [unwired: 1 in, 1 out]
            n74 = call <vilib>:"Add State(s) to Queue__jki_lib_state_machine.vi"("State(s) in Front (\"\")"="Macro: Exit", "State(s) in (\"\")"=w148) -> ("States Out"=w147:string)  [unwired: 13 in]
            n75 = event-data("Discard?"=TRUE) -> ()  [unwired: 1 in, 1 out]
          }
        }
      }
      frame "---------- Core ----------" {
        # "Do not put any code in this frame.\n(it is a separator no-op)"
        n76 = call <vilib>:"Add State(s) to Queue__jki_lib_state_machine.vi"("State(s) in (\"\")"=w152) -> ("States Out"=w151:string)  [unwired: 14 in]
      }
      frame Default {
        w162 = 42 items=["No error", "Argument error", "Memory is full", "Out of zone", "End of file", "File already open", "Generic file I/O error", "File not found", "File permission error", "Disk is full", "Duplicate path", "Too many files open", "System feature not enabled", "Resource file not found", "Cannot add resource", "Resource not found", "Image not found", "Image memory error", "Pen does not exist", "Config type invalid", "Config token not found", "Config parse error", "Config memory error", "Bad external code format", "Bad external code offset", "External code not present", "Null window", "Destroy window error", "Null menu", "Print aborted", "Bad print record", "Print driver error", "Windows error during printing", "Memory error during printing", "Print dialog error", "Generic print error", "Invalid device refnum", "Device not found", "Device parameter error", "Device unit error", "Cannot open device", "Device call aborted", "Generic error", "Cancelled by user", "Object ID too low", "Object ID too high", "Object not in heap", "Unknown heap", "Unknown object (invalid DefProc)", "Unknown object (DefProc not in table)", "Message out of range", "Invalid (null) method", "Unknown message", "Manager call not supported", "Bad address", "Network operation in progress", "Network operation timed out", "Connection is busy", "Network attribute not supported", "Network error", "Address in use", "System out of memory", "Connection aborted", "Connection refused", "Not connected", "Already connected", "Connection closed", "Initialization error (interapplication manager)", "Bad occurrence", "Wait on unbound occurrence handler", "Occurrence queue overflow", "Datalog type conflict", "Unused", "Unrecognized type (interapplication manager)", "Memory corrupt", "Failed to make temporary DLL", "Old CIN version", "Drag socket not found", "Failed to load drop-object", "Failed to register OLE object", "Failed to release OLE object", "Format specifier type mismatch", "Unknown format specifier", "Too few format specifiers", "Too many format specifiers", "Scan failed", "Newer CIN version", "Error converting to variant", "Runtime menu error", "Password tampered", "Variant attribute not found", "Incompatible variant data type", "Event data is not available", "Event Store is not present", "Occurrence is not found", "Event Queue is not created", "Event info is not available", "Refnum passed is NULL", "Error retrieving Class GUID", "Error retrieving CoClass GUID", "Error retrieving TypeLib GUID.", "Bad built application magic bytes.", "Specific driver is different from the specific driver associated with the Logical Name.", "There is no session opened to the class driver.", "Max Error", "MAX - Error with config objects", "MAX - Error loading configuration", "MAX - Group not supported"]
        # "Current State"
        # "Do not delete, rename, or modify this frame.\n(this is used to capture unhandled states and typos)"
        # "Handle mistyped state name (developer tool)"
        n77 = Format Into String(format string="Software Exception: Unhandled State \"%s\"." ("message"), error in=w158, w153) -> (resulting string=w161:string, error out=w160:errorcluster)  [unwired: 1 in]
        n78 = call <vilib>:"Error Cluster From Error Code.vi"("show call chain? (False)"=TRUE, "error in (no error)"=w160, "error message (\"\")"=w161, "error code (0)"=w162) -> ("error out"=w159:errorcluster)  [unwired: 5 in]
        n79 = call <vilib>:"Add State(s) to Queue__jki_lib_state_machine.vi"("State(s) in (\"\")"=w157) -> ("States Out"=w156:string)  [unwired: 14 in]
      }
      frame "Initialize Core Data" {
        # "Do not delete, rename, or modify this frame.\n(this is used to determine panel behavior on exit)"
        # "originally closed?"
        # "exe?"
        # "If panel starts closed or is an EXE, then close it when we exit"
        n80 = property class="VI"() -> ("FP.State"=w166:T4)  [unwired: 2 in, 2 out]
        n81 = property class="App"() -> ("App.Kind"=w172:T5)  [unwired: 2 in, 2 out]
        n82 = control-ref of="Current VI Reference"() -> (w167:refnum<vi>)
        n83 = Equal?(x=w166, y=T4."Closed" ("Front Panel Window:State")) -> (x = y?=w164:bool)
        n84 = Equal?(x=w172, y=T5."Run Time System" ("Application:Kind")) -> (x = y?=w170:bool)
        n85 = Or(x=w164, y=w170) -> (x .or. y?=w168:bool)
        n86 = Bundle By Name(cluster=w169, "Core.Current VI Reference"=w167, "Core.Close Panel on Exit?"=w168) -> (w174:T6)
        n87 = call <vilib>:"Add State(s) to Queue__jki_lib_state_machine.vi"("State(s) in (\"\")"=w176) -> ("States Out"=w175:string)  [unwired: 14 in]
      }
      frame "Error Handler" {
        # "Unhandled Error -- Display it"
        # "Handle any errors here.\nYou can also output any states to clean-up after errors occur"
        # "Clear error"
        n88 = call <vilib>:"General Error Handler.vi"("error in (no error)"=w178) -> ()  [unwired: 10 in, 5 out]
        n89 = call <vilib>:"Add State(s) to Queue__jki_lib_state_machine.vi"("State(s) in Front (\"\")"="/* Post Error States", "State(s) in (\"\")"=w182) -> ("States Out"=w181:string)  [unwired: 13 in]
      }
      frame "Exit" {
        # "Do not put any code in this frame.\n(No errors that occur here will be handled.)"
        n90 = call <vilib>:"Add State(s) to Queue__jki_lib_state_machine.vi"("State(s) in (\"\")"=w187) -> ("States Out"=w186:string)  [unwired: 14 in]
      }
      frame "---------- Data ----------" {
        # "Do not put any code in this frame.\n(It is a separator no-op. You can make a copy of this frame to create a new Data frame)"
        n91 = call <vilib>:"Add State(s) to Queue__jki_lib_state_machine.vi"("State(s) in (\"\")"=w191) -> ("States Out"=w190:string)  [unwired: 14 in]
      }
      frame "Data: Initialize" {
        w203 = T8 {"Current VI Reference"=refnum, "Close Panel on Exit?"=FALSE}  # Core
        w205 = TRUE  # Your Boolean data
        w204 = ""  # String
        # "do not delete - used by framework"
        # "Add new data here."
        # "Data names and types of shift register data are defined by this bundle."
        # "Initialize the shift-register data, here.\n(data names are defined by what you wire into the bundle function)"
        n92 = local read "Preset Table Control"() -> (w201:string[][])
        n93 = property on="Headers" class="Tbl (strict)"() -> ("Column Headers[]"=w202:string[])  [unwired: 2 in, 2 out]
        n94 = local read "Queue Table Control"() -> (w200:string[][])
        n95 = call "PresetExecutionDataCluster.vi"() -> ("Preset Manager Cluster"=w199:T9)  [unwired: 1 in]
        n96 = Bundle("Core"=w203, "Your Boolean data"=w205, "String"=w204, "Preset Table Control"=w201, "Column Headers[]"=w202, "Queue Table Control"=w200, "Preset Manager Cluster"=w199) -> (w198:T6)  [unwired: 1 in]
        n97 = call <vilib>:"Add State(s) to Queue__jki_lib_state_machine.vi"("State(s) in (\"\")"=w208) -> ("States Out"=w207:string)  [unwired: 14 in]
        n98 = Bundle By Name(cluster=w198, "Preset Manager Cluster.DevStatusQueue"="DevStatusQueue", "Preset Manager Cluster.Experiment Name"="Experiment Name", "Preset Manager Cluster.Software Root"="Software Root", "Preset Manager Cluster.Filtered Devices List"="Filtered Devices List", "Preset Manager Cluster.Virtual Devices List"="Virtual Devices List") -> (w197:T6)
      }
      frame "Data: Cleanup" {
        # "Cleanup any data and references, here.\n(this is called automatically, by the Macro: Exit)"
        n99 = Unbundle By Name(w209) -> ("Core.Current VI Reference"=w212:refnum<vi>)
        n100 = Close Reference(reference=w212, error in (no error)=w211) -> (error out=w210:errorcluster)
        n101 = call <vilib>:"Add State(s) to Queue__jki_lib_state_machine.vi"("State(s) in (\"\")"=w214) -> ("States Out"=w213:string)  [unwired: 14 in]
      }
      frame "---------- UI ----------" {
        # "Do not put any code in this frame.\n(It is a separator no-op. You can make a copy of this frame to create a new UI frame)"
        n102 = call <vilib>:"Add State(s) to Queue__jki_lib_state_machine.vi"("State(s) in (\"\")"=w218) -> ("States Out"=w217:string)  [unwired: 14 in]
      }
      frame "UI: Initialize" {
        # "Initialize the User Interface, here.\n(this is called automatically, by the Macro: Init)"
        n103 = call <vilib>:"Add State(s) to Queue__jki_lib_state_machine.vi"("State(s) in (\"\")"=w222) -> ("States Out"=w221:string)  [unwired: 14 in]
      }
      frame "UI: Cursor Set" {
        # "Argument"
        # "Set and Unset Cursor Busy.\n(Usage: \"UI: Cursor Set >> Busy|Idle\")"
        n104 = case shown="\"Idle\", Default" w223 {
          tunnel: w225 -> [w230 w232]
          tunnel: [w229 w231] -> w224
          frame "Idle", Default {
            n105 = call <vilib>:"Unset Busy.vi"("error in (no error)"=w230) -> ("error out"=w229:errorcluster)  [unwired: 10 in]
          }
          frame "Busy" {
            n106 = call <vilib>:"Set Busy.vi"("error in (no error)"=w232) -> ("error out"=w231:errorcluster)  [unwired: 9 in, 1 out]
          }
        }
        n107 = call <vilib>:"Add State(s) to Queue__jki_lib_state_machine.vi"("State(s) in (\"\")"=w228) -> ("States Out"=w227:string)  [unwired: 14 in]
      }
      frame "UI: Front Panel State" {
        # "Argument"
        # "Set Front Panel Open or Closed\n(Usage: \"UI: Front Panel State >> Open|Close\")"
        n108 = Unbundle By Name(w235) -> ("Core.Current VI Reference"=w234:refnum<vi>)
        n109 = case shown="\"Minimize\", \"Minimized\"" w233 {
          tunnel: w237 -> [w245 w260 w271 w284 w297]
          tunnel: [w247 w261 w273 w286 w299] -> w236
          tunnel: w234 -> [w246 w258 w272 w285 w298]
          frame "Open", "Standard", Default {
            w240 = T4."Standard" ("State")
            n110 = property class="VI"(reference=w246, error in=w245) -> (reference out=w243:refnum<vi>, error out=w244:errorcluster, "FP.State"=w242:T4)
            n111 = Not Equal?(x=w242, y=w240) -> (x != y?=w241:bool)
            n112 = case shown="True" w241 {
              tunnel: [w251 w253] -> w247
              tunnel: w244 -> [w250 w253]
              tunnel: w243 -> [w249 _]
              tunnel: w240 -> [w248 _]
              frame True {
                n113 = invoke class="VI" method="FP.Open"(reference=w249, error in=w250, "Activate"=TRUE, "State"=w248) -> (error out=w251:errorcluster)  [unwired: 1 in, 4 out]
              }
              frame False {
              }
            }
          }
          frame "Close", "Closed" {
            n114 = property class="VI"(reference=w258, error in=w260) -> (reference out=w257:refnum<vi>, error out=w259:errorcluster, "FP.State"=w255:T4)
            n115 = Not Equal?(x=w255, y=T4."Closed" ("Front Panel Window:State")) -> (x != y?=w254:bool)
            n116 = case shown="True" w254 {
              tunnel: [w262 w265] -> w261
              tunnel: w259 -> [w262 w264]
              tunnel: w257 -> [_ w263]
              frame False {
              }
              frame True {
                n117 = invoke class="VI" method="FP.Close"(reference=w263, error in=w264) -> (error out=w265:errorcluster)  [unwired: 1 in, 2 out]
              }
            }
          }
          frame "Hidden", "Hide" {
            w266 = T4."Hidden" ("State")
            n118 = property class="VI"(reference=w272, error in=w271) -> (reference out=w269:refnum<vi>, error out=w270:errorcluster, "FP.State"=w268:T4)
            n119 = Not Equal?(x=w268, y=w266) -> (x != y?=w267:bool)
            n120 = case shown="True" w267 {
              tunnel: [w277 w278] -> w273
              tunnel: w270 -> [w276 w278]
              tunnel: w269 -> [w275 _]
              tunnel: w266 -> [w274 _]
              frame True {
                n121 = invoke class="VI" method="FP.Open"(reference=w275, error in=w276, "State"=w274) -> (error out=w277:errorcluster)  [unwired: 2 in, 4 out]
              }
              frame False {
              }
            }
          }
          frame "Minimize", "Minimized" {
            w279 = T4."Minimized" ("State")
            n122 = property class="VI"(reference=w285, error in=w284) -> (reference out=w282:refnum<vi>, error out=w283:errorcluster, "FP.State"=w281:T4)
            n123 = Not Equal?(x=w281, y=w279) -> (x != y?=w280:bool)
            n124 = case shown="True" w280 {
              tunnel: [w290 w291] -> w286
              tunnel: w283 -> [w289 w291]
              tunnel: w282 -> [w288 _]
              tunnel: w279 -> [w287 _]
              frame True {
                n125 = invoke class="VI" method="FP.Open"(reference=w288, error in=w289, "State"=w287) -> (error out=w290:errorcluster)  [unwired: 2 in, 4 out]
              }
              frame False {
              }
            }
          }
          frame "Maximize", "Maximized" {
            w292 = T4."Maximized" ("State")
            n126 = property class="VI"(reference=w298, error in=w297) -> (reference out=w295:refnum<vi>, error out=w296:errorcluster, "FP.State"=w294:T4)
            n127 = Not Equal?(x=w294, y=w292) -> (x != y?=w293:bool)
            n128 = case shown="True" w293 {
              tunnel: [w303 w304] -> w299
              tunnel: w296 -> [w302 w304]
              tunnel: w295 -> [w301 _]
              tunnel: w292 -> [w300 _]
              frame True {
                n129 = invoke class="VI" method="FP.Open"(reference=w301, error in=w302, "State"=w300) -> (error out=w303:errorcluster)  [unwired: 2 in, 4 out]
              }
              frame False {
              }
            }
          }
        }
        n130 = call <vilib>:"Add State(s) to Queue__jki_lib_state_machine.vi"("State(s) in (\"\")"=w239) -> ("States Out"=w238:string)  [unwired: 14 in]
      }
      frame "---------- Macro ----------" {
        # "Do not put any code in this frame.\n(It is a separator no-op. You can make a copy of this frame to create a new Macro frame)"
        n131 = call <vilib>:"Add State(s) to Queue__jki_lib_state_machine.vi"("State(s) in (\"\")"=w308) -> ("States Out"=w307:string)  [unwired: 14 in]
      }
      frame "Macro: Initialize" {
        w312 = 0
        w311 = string[][] [] ("Queue Table")
        w315 = "Data: Initialize\nInitialize Core Data\nUI: Initialize\nUI: Front Panel State >> Open\nInitialize UDP Variables"  # Data: Initialize Initialize Core Data UI: Initialize UI: Front Panel State >> Open Initialize UDP Variables
        # "Initialization Macro\n(This is called once, when the VI starts)"
        n132 = property on="Queue Element" class="DigNum (strict)"("Value"=w312) -> ()  [unwired: 2 in, 2 out]
        n133 = property on="Queue Table" class="Tbl (strict)"("Value"=w311) -> ()  [unwired: 2 in, 2 out]
        n134 = property on="Queue Size" class="DigNum (strict)"("Value"=w312) -> ()  [unwired: 2 in, 2 out]
        n135 = property on="Preset Table Control" class="Tbl (strict)"("Value"=w311) -> ()  [unwired: 2 in, 2 out]
        n136 = property on="Preset Devices Not in Experiment" class="LstBox (strict)"("Item Names"=string[] [] ("Queue Table")) -> ()  [unwired: 2 in, 2 out]
        n137 = call <vilib>:"Add State(s) to Queue__jki_lib_state_machine.vi"("State(s) in Front (\"\")"=w315, "State(s) in (\"\")"=w319) -> ("States Out"=w318:string)  [unwired: 13 in]
        n138 = property on="Preset Execution Indicator" class="Bool (strict)"("Blinking"=FALSE, "Caption.Text"="" ("Boolean Text.Text"), "Colors [4]"=cluster{u32, u32}[] [{32639, 0}]) -> ()  [unwired: 2 in, 2 out]
      }
      frame "Macro: Exit" {
        # "Exit Macro\n(This is called once, when the VI exits)"
        n139 = Unbundle By Name(w326) -> ("Core.Close Panel on Exit?"=w325:bool)
        n140 = Select(t="UI: Front Panel State >> Close", s=w325, f="") -> (s? t:f=w322:string)
        n141 = call <vilib>:"Add State(s) to Queue__jki_lib_state_machine.vi"("State(s) in (\"\")"=w322, "State(s) at Back (\"\")"="Data: Cleanup\nExit") -> ("States Out"=w320:string)  [unwired: 13 in]
        n142 = call <vilib>:"Add State(s) to Queue__jki_lib_state_machine.vi"("State(s) in Front (\"\")"=w320, "State(s) in (\"\")"=w329) -> ("States Out"=w328:string)  [unwired: 13 in]
      }
      frame "Initialize UDP Variables" {
        # "Do not put any code in this frame.\n(It is a separator no-op. You can make a copy of this frame to create a new Macro frame)"
        n143 = Unbundle By Name(w338) -> ("Preset Manager Cluster.Experiment Name"=w336:string)
        n144 = call "UPD Variable Init.vi"("Expt Name"=w336) -> ("Mcast Address"=w332:string, "UDP timeout ms"=w333:i32, "MC Multicast"=w334:refnum<k16>, "My IP"=w335:string, "Mcast remote"=w331:u16, "> Name, devtype, ip, dev comm port, class, location for all devices>"=w330:string[][])  [unwired: 5 in]
        n145 = call <vilib>:"Add State(s) to Queue__jki_lib_state_machine.vi"("State(s) in (\"\")"=w341) -> ("States Out"=w340:string)  [unwired: 14 in]
        n146 = Bundle By Name(cluster=w338, "Preset Manager Cluster.My IP"=w335, "Preset Manager Cluster.MC Multicast"=w334, "Preset Manager Cluster.UDP timeout ms"=w333, "Preset Manager Cluster.Mcast address"=w332, "Preset Manager Cluster.MCast Remote"=w331, "Preset Manager Cluster.All Devices Core Info"=w330) -> (w337:T6)
      }
      frame "---------- Menu Control ----------" {
        # "Template Separator\n(You can make a copy of, or modify, this frame)"
        n147 = call <vilib>:"Add State(s) to Queue__jki_lib_state_machine.vi"("State(s) in (\"\")"=w345) -> ("States Out"=w344:string)  [unwired: 14 in]
      }
      frame "Compare Table" {
        # "Template Separator\n(You can make a copy of, or modify, this frame)"
        n148 = property on="PRESET FROM DB" class="Tbl (strict)"() -> ("Value"=w352:string[][])  [unwired: 2 in, 2 out]
        n149 = property on="ECS File" class="Tbl (strict)"() -> ("Value"=w351:string[][])  [unwired: 2 in, 2 out]
        n150 = call "Left Join.vi"("Array 2"=w351, "Array 1"=w352) -> ("Left Joined Array"=w349:string[][])  [unwired: 9 in]
        n151 = call <vilib>:"Add State(s) to Queue__jki_lib_state_machine.vi"("State(s) in Front (\"\")"="Table Update" ("State(s) in Front (\"\")"), "State(s) in (\"\")"=w355) -> ("States Out"=w354:string)  [unwired: 13 in]
        n152 = Bundle By Name(cluster=w350, "Preset Table Control"=w349, "Column Headers[]"=string[] ["Device Name", "Device Variable", "Preset Value", "ECS Value"] ("Column Headers")) -> (w348:T6)
      }
      frame "Choose Values" {
        # "Template Separator\n(You can make a copy of, or modify, this frame)"
        n153 = property on="Preset Table Control" class="Tbl (strict)"() -> ("Value"=w359:string[][])  [unwired: 2 in, 2 out]
        n154 = call "Value_Selection_in_Table_GUI.vi"("Column Headers"=string[] ["Device Name", "Device Variable", "Preset Value", "ECS Value"], "SELECTION TABLE - Click on values to keep"=w359) -> ("Coordinate Array"=→"Coordinate Array":i32[][])  [unwired: 9 in]
        n155 = call <vilib>:"Add State(s) to Queue__jki_lib_state_machine.vi"("State(s) in Front (\"\")"="Implement Value Change" ("State(s) in Front (\"\")"), "State(s) in (\"\")"=w363) -> ("States Out"=w362:string)  [unwired: 13 in]
      }
      frame "Implement Value Change" {
        # "Template Separator\n(You can make a copy of, or modify, this frame)"
        n156 = Unbundle By Name(w369) -> ("Preset Table Control"=w367:string[][])
        n157 = property on="Coordinate Array" class="Arr (strict)"() -> ("Value"=w366:i32[][])  [unwired: 2 in, 2 out]
        n158 = call "Value_Update_to_Preset.vi"("Coordinate Array with Changes"=w366, "Input Table"=w367) -> ("Column Headers"=w364:string[], "Output Table with Changes"=w365:string[][])  [unwired: 8 in]
        n159 = Bundle By Name(cluster=w369, "Preset Table Control"=w365, "Column Headers[]"=w364) -> (w368:T6)
        n160 = call <vilib>:"Add State(s) to Queue__jki_lib_state_machine.vi"("State(s) in Front (\"\")"="Table Update" ("State(s) in Front (\"\")"), "State(s) in (\"\")"=w373) -> ("States Out"=w372:string)  [unwired: 13 in]
      }
      frame "Load Preset from DB" {
        # "Template Separator\n(You can make a copy of, or modify, this frame)"
        n161 = property on="Preset Menu" class="Ring (strict)"() -> ("RingText.Text"=w374:string)  [unwired: 2 in, 2 out]
        n162 = call "Preset_to_Array.vi"("Preset Name"=w374) -> ("Column Headers"=w376:string[], "Preset Table"=w375:string[][])  [unwired: 9 in]
        "PRESET FROM DB" <- w375
        n163 = Bundle By Name(cluster=w379, "Preset Table Control"=w375, "Column Headers[]"=w376, "Preset Manager Cluster.PresetName"=w374) -> (w378:T6)
        n164 = call <vilib>:"Add State(s) to Queue__jki_lib_state_machine.vi"("State(s) in Front (\"\")"="Table Update\nExpt Device Check>>Preset Only" ("State(s) in Front (\"\")"), "State(s) in (\"\")"=w382) -> ("States Out"=w381:string)  [unwired: 13 in]
      }
      frame "Load Configuration File" {
        # "Template Separator\n(You can make a copy of, or modify, this frame)"
        n165 = call "Configuration_to_Array.vi"("file (use dialog)"="Navigate to ECS File") -> ("Table Control"=w385:string[][])  [unwired: 10 in]
        "ECS File" <- w385
        n166 = Bundle By Name(cluster=w387, "Preset Table Control"=w385, "Column Headers[]"=string[] ["Device Name", "Device Variable", "ECS Values"] ("Column Headers")) -> (w386:T6)
        n167 = call <vilib>:"Add State(s) to Queue__jki_lib_state_machine.vi"("State(s) in Front (\"\")"="Table Update" ("State(s) in Front (\"\")"), "State(s) in (\"\")"=w391) -> ("States Out"=w390:string)  [unwired: 13 in]
      }
      frame "Save Preset" {
        # "Template Separator\n(You can make a copy of, or modify, this frame)"
        n168 = call <vilib>:"Three Button Dialog.vi"("Right Button Text (\"Cancel\")"="Cancel" ("Right Button Text (\"Cancel\")"), "Center Button Text (\"No\")"="Overwrite Existing Preset" ("Right Button Text (\"Cancel\")"), "Left Button Text (\"Yes\")"="Save as New Preset" ("Left Button Text (\"Yes\")"), "message"="Save the current preset as - ") -> ("Which Button?"=w393:T10)  [unwired: 7 in]
        n169 = case shown="\"Right Button\", Default" w393 {
          tunnel: ["Save as New Preset" ("State(s) in Front (\"\")") "Overwrite Existing Preset" ("Right Button Text (\"Cancel\")") _] -> w392
          frame "Left Button" {
          }
          frame "Center Button" {
          }
          frame "Right Button", Default {
          }
        }
        n170 = call <vilib>:"Add State(s) to Queue__jki_lib_state_machine.vi"("State(s) in Front (\"\")"=w392, "State(s) in (\"\")"=w401) -> ("States Out"=w400:string)  [unwired: 13 in]
      }
      frame "Save as New Preset" {
        # "Template Separator\n(You can make a copy of, or modify, this frame)"
        n171 = call "Preset Name"() -> ("Name"=w405:string, "OK"=w414:bool)  [unwired: 17 in, 1 out]
        n172 = property on="Preset Menu" class="Ring (strict)"() -> ("Strings []"=w411:string[])  [unwired: 2 in, 2 out]
        n173 = Search 1D Array(1D array=w411, element=w405) -> (index of element=w410:i32)  [unwired: 1 in]
        n174 = call <vilib>:"Trim Whitespace.vi"("string"=w405) -> ("trimmed string"=w413:string)  [unwired: 1 in]
        n175 = Equal?(x=w413, y="") -> (x = y?=w408:bool)
        n176 = Not Equal?(x=w410, y=-1) -> (x != y?=w407:bool)
        n177 = Or(x=w408, y=w407) -> (x .or. y?=w406:bool)
        n178 = case shown="True" w414 {
          tunnel: w406 -> [_ w420]
          tunnel: w405 -> [_ w419]
          frame False {
          }
          frame True {
            n179 = case shown="False" w420 {
              tunnel: w419 -> [w421 _]
              frame False {
                n180 = stacked-sequence {
                  tunnel: w421 -> [w423]
                  frame #0 {
                    n181 = local read "Preset Table Control"() -> (w422:string[][])
                    n182 = for {
                      tunnel: w423 -> [w428]
                      tunnel: w422 -> [w424] mode=indexing
                      n183 = Insert Into Array(array=w424, index=0, new element=w428) -> (w426:string[])
                      n184 = call "SQL Insert null.vi"("Values"=w426, "Column Names"=string[] ["presetName", "presetDevice", "presetVariable", "presetValue"], "Table"="Presets") -> ("Query String"=w425:string)  [unwired: 8 in]
                      n185 = disable-structure shown="Enabled" {
                        disable-tunnel: w425 -> [w431 _]
                        frame Enabled {
                          n186 = call "SQL Server Info.vi"() -> ("SQL Server Info"=w432:T12)
                          n187 = call "SQL Query.vi"("SQL Server Info"=w432, "Query"=w431) -> ()  [unwired: 8 in, 2 out]
                        }
                        frame Disabled {
                        }
                      }
                    }
                  }
                }
              }
              frame True {
                n188 = One Button Dialog(message="Name field was blank or the Preset Name already exists") -> ()  [unwired: 1 in, 1 out]
              }
            }
          }
        }
        n189 = call <vilib>:"Add State(s) to Queue__jki_lib_state_machine.vi"("State(s) in Front (\"\")"="Load Preset from DB>>Table Update" ("State(s) in Front (\"\")"), "State(s) in (\"\")"=w418) -> ("States Out"=w417:string)  [unwired: 13 in]
      }
      frame "Overwrite Existing Preset" {
        # "Template Separator\n(You can make a copy of, or modify, this frame)"
        n190 = property on="Preset Menu" class="Ring (strict)"() -> ("RingText.Text"=w435:string)  [unwired: 2 in, 2 out]
        n191 = Concatenate Strings("Are you sure you want to overwrite " ("string"), w435, " with the current table ?" ("string")) -> (w438:string)
        n192 = Two Button Dialog(message=w438, 2:"Yes" ("T button name (\"OK\")")) -> (T button?=w436:bool)  [unwired: 1 in]
        n193 = case shown="True" w436 {
          tunnel: w435 -> [_ w445]
          frame False {
          }
          frame True {
            n194 = stacked-sequence {
              seq-local: [w446 _] -> [_ w456]
              tunnel: w445 -> [w447 w455]
              tunnel: [_ w456] -> _
              frame #0 {
                n195 = disable-structure shown="Enabled" {
                  disable-tunnel: w447 -> [w451 _]
                  disable-tunnel: [w448 _] -> w446
                  frame Enabled {
                    n196 = Concatenate Strings("DELETE FROM Presets WHERE presetName='", w451, "'" ("string")) -> (w449:string)
                    n197 = call "SQL Server Info.vi"() -> ("SQL Server Info"=w453:T12)
                    n198 = call "SQL Query.vi"("SQL Server Info"=w453, "Query"=w449) -> ("error out"=w448:errorcluster)  [unwired: 8 in, 1 out]
                  }
                  frame Disabled {
                  }
                }
              }
              frame #1 {
                n199 = local read "Preset Table Control"() -> (w454:string[][])
                n200 = for {
                  tunnel: w456 -> [w464]
                  tunnel: w455 -> [w461]
                  tunnel: w454 -> [w457] mode=indexing
                  n201 = Insert Into Array(array=w457, index=0, new element=w461) -> (w459:string[])
                  n202 = call "SQL Insert null.vi"("Values"=w459, "Column Names"=string[] ["presetName", "presetDevice", "presetVariable", "presetValue"], "Table"="Presets") -> ("Query String"=w458:string)  [unwired: 8 in]
                  n203 = disable-structure shown="Enabled" {
                    disable-tunnel: w464 -> [w466 _]
                    disable-tunnel: w458 -> [w465 _]
                    frame Enabled {
                      n204 = call "SQL Server Info.vi"() -> ("SQL Server Info"=w467:T12)
                      n205 = call "SQL Query.vi"("error in (no error)"=w466, "SQL Server Info"=w467, "Query"=w465) -> ()  [unwired: 7 in, 2 out]
                    }
                    frame Disabled {
                    }
                  }
                }
              }
            }
          }
        }
        n206 = call <vilib>:"Add State(s) to Queue__jki_lib_state_machine.vi"("State(s) in Front (\"\")"="Load Preset from DB>>Table Update" ("State(s) in Front (\"\")"), "State(s) in (\"\")"=w444) -> ("States Out"=w443:string)  [unwired: 13 in]
      }
      frame "Delete Preset" {
        # "Template Separator\n(You can make a copy of, or modify, this frame)"
        n207 = property on="Preset Menu" class="Ring (strict)"() -> ("RingText.Text"=w468:string)  [unwired: 2 in, 2 out]
        n208 = Concatenate Strings("Are you sure you want to delete " ("string"), w468, ". NOTE - THIS ACTION IS NOT REVERSIBLE" ("string")) -> (w471:string)
        n209 = Two Button Dialog(message=w471, 2:"Yes" ("T button name (\"OK\")")) -> (T button?=w469:bool)  [unwired: 1 in]
        n210 = case shown="True" w469 {
          tunnel: w468 -> [_ w479]
          frame False {
          }
          frame True {
            n211 = stacked-sequence {
              tunnel: w479 -> [w480]
              frame #0 {
                n212 = disable-structure shown="Enabled" {
                  disable-tunnel: w480 -> [w485 _]
                  frame Enabled {
                    n213 = Concatenate Strings("DELETE FROM Presets WHERE presetName='", w485, "'" ("string")) -> (w481:string)
                    n214 = call "SQL Server Info.vi"() -> ("SQL Server Info"=w484:T12)
                    n215 = call "SQL Query.vi"("SQL Server Info"=w484, "Query"=w481) -> ()  [unwired: 8 in, 2 out]
                  }
                  frame Disabled {
                  }
                }
              }
            }
          }
        }
        n216 = call <vilib>:"Add State(s) to Queue__jki_lib_state_machine.vi"("State(s) in Front (\"\")"="Load Preset from DB>>Table Update" ("State(s) in Front (\"\")"), "State(s) in (\"\")"=w478) -> ("States Out"=w477:string)  [unwired: 13 in]
      }
      frame "Execute Preset" {
        # "Template Separator\n(You can make a copy of, or modify, this frame)"
        n217 = control-ref of="Preset Execution Indicator"() -> (w489:refnum<vi>)
        n218 = property on="Property Node" class="Bool (strict)"(reference=w489, "Blinking"=TRUE, "Caption.Text"="Executing Preset" ("Boolean Text.Text")) -> ()  [unwired: 1 in, 2 out]
        n219 = call <vilib>:"Add State(s) to Queue__jki_lib_state_machine.vi"("State(s) in Front (\"\")"="Send Preset Command" ("State(s) in Front (\"\")"), "State(s) in (\"\")"=w493) -> ("States Out"=w492:string)  [unwired: 13 in]
      }
      frame "-------Table Update--------" {
        # "Template Separator\n(You can make a copy of, or modify, this frame)"
        n220 = call <vilib>:"Add State(s) to Queue__jki_lib_state_machine.vi"("State(s) in (\"\")"=w497) -> ("States Out"=w496:string)  [unwired: 14 in]
      }
      frame "Table Update" {
        # "Template Separator\n(You can make a copy of, or modify, this frame)"
        n221 = Unbundle By Name(w500) -> ("Preset Table Control"=w499:string[][], "Column Headers[]"=w498:string[])
        n222 = call <vilib>:"Add State(s) to Queue__jki_lib_state_machine.vi"("State(s) in (\"\")"=w503) -> ("States Out"=w502:string)  [unwired: 14 in]
        n223 = property on="Preset Table Control" class="Tbl (strict)"("Value"=w499, "Column Headers[]"=w498) -> ()  [unwired: 2 in, 2 out]
      }
      frame "--------Queue Presets------------" {
        # "Template Separator\n(You can make a copy of, or modify, this frame)"
        n224 = call <vilib>:"Add State(s) to Queue__jki_lib_state_machine.vi"("State(s) in (\"\")"=w507) -> ("States Out"=w506:string)  [unwired: 14 in]
      }
      frame "Init: Queue Preset" {
        # "Template Separator\n(You can make a copy of, or modify, this frame)"
        n225 = property on="Tab Control" class="TabCtl (strict)"() -> ("Value"=w508:T1)  [unwired: 2 in, 2 out]
        n226 = Equal?(x=w508, y=1) -> (x = y?=w511:bool)
        n227 = case shown="False" w511 {
          frame False {
          }
          frame True {
            n228 = call "preset SQL Queries.vi"("Preset Query"=Preset_Query_Enum."GetAllPresetNames") -> ("data"=w515:string[][])  [unwired: 8 in, 2 out]
            n229 = Array Subset(array=w515, index (row)=1 ("index")) -> (w516:string[][])  [unwired: 3 in]
            n230 = property on="Queue Table Control" class="Tbl (strict)"("Value"=w516) -> ()  [unwired: 2 in, 2 out]
          }
        }
        n231 = call <vilib>:"Add State(s) to Queue__jki_lib_state_machine.vi"("State(s) in (\"\")"=w514) -> ("States Out"=w513:string)  [unwired: 14 in]
      }
      frame "Reset Queue" {
        # "Template Separator\n(You can make a copy of, or modify, this frame)"
        n232 = property on="Queue Table" class="Tbl (strict)"("Value"=string[][] [] ("Queue Table")) -> ()  [unwired: 2 in, 2 out]
        n233 = call <vilib>:"Add State(s) to Queue__jki_lib_state_machine.vi"("State(s) in (\"\")"=w523) -> ("States Out"=w522:string)  [unwired: 14 in]
      }
      frame "Execute Queue" {
        # "Template Separator\n(You can make a copy of, or modify, this frame)"
        n234 = flat-sequence {
          frame #0 {
            w529 = TRUE
            n235 = property on="Queue Size" class="DigNum (strict)"("Visible"=w529) -> ()  [unwired: 2 in, 2 out]
            n236 = property on="Current Preset Queue Element" class="Str"("Visible"=w529) -> ()  [unwired: 2 in, 2 out]
            n237 = property on="Queue Progress Bar" class="Slide (strict)"("Visible"=w529) -> ()  [unwired: 2 in, 2 out]
          }
          frame #1 {
            n238 = property on="Queue Table" class="Tbl (strict)"() -> ("Value"=w537:string[][])  [unwired: 2 in, 2 out]
            n239 = property on="Using Queue" class="Bool (strict)"("Val(Sgnl)"=TRUE ("Value (Signaling)")) -> ()  [unwired: 2 in, 2 out]
            n240 = property on="Queue Progress Bar" class="Slide (strict)"("Value"=u8 0 ("Queue Progress Bar"), "Maximum"=1.0 ("Data Entry Limits:Maximum")) -> ()  [unwired: 2 in, 2 out]
            n241 = Index Array(array=w537, index (col)=0 ("disabled index (col)")) -> (element=w535:string[])  [unwired: 1 in]
            n242 = Array Size(array=w535) -> (size(s)=→"Queue Size":i32)
            "Queue Element" <- 1 ("Element")
          }
          frame #2 {
          }
        }
        n243 = call <vilib>:"Add State(s) to Queue__jki_lib_state_machine.vi"("State(s) in Front (\"\")"="Preset Queue Loading" ("State(s) in Front (\"\")"), "State(s) in (\"\")"=w528) -> ("States Out"=w527:string)  [unwired: 13 in]
      }
      frame "Preset Queue Loading" {
        # "Template Separator\n(You can make a copy of, or modify, this frame)"
        n244 = flat-sequence {
          tunnel: w539 -> [w547]
          tunnel: [w548] -> w540
          tunnel: [w546] -> w538
          frame #0 {
            n245 = property on="Queue Element" class="DigNum (strict)"() -> ("Value"=w545:i32)  [unwired: 2 in, 2 out]
            n246 = property on="Queue Size" class="DigNum (strict)"() -> ("Value"=w544:i32)  [unwired: 2 in, 2 out]
            n247 = Less?(x=w544, y=w545) -> (x < y?=w549:bool)
            n248 = case shown="False" w549 {
              tunnel: [w555 ""] -> w548
              tunnel: w547 -> [w554 w565]
              tunnel: [w553 w565] -> w546
              tunnel: w545 -> [w552 _]
              tunnel: w544 -> [w551 _]
              frame False {
                n249 = Divide(x=w552, y=w551) -> (x/y=w550:dbl)
                n250 = flat-sequence {
                  tunnel: w554 -> [w558]
                  tunnel: [w557] -> w553
                  tunnel: ["Execute Preset"] -> w555
                  frame #0 {
                    n251 = property on="Queue Element" class="DigNum (strict)"() -> ("Value"=w560:i32)  [unwired: 2 in, 2 out]
                    n252 = local read "Queue Table"() -> (w562:string[][])
                    n253 = Decrement(x=w560) -> (x-1=w559:i32)
                    n254 = Index Array(array=w562, index (row)=w559, index (col)=0 ("disabled index (col)")) -> (element=w556:string)
                    "Current Preset Queue Element" <- w556
                    n255 = Bundle By Name(cluster=w558, "Preset Manager Cluster.PresetName"=w556) -> (w557:T6)
                  }
                  frame #1 {
                  }
                }
                n256 = property on="Queue Progress Bar" class="Slide (strict)"("Value"=w550) -> ()  [unwired: 2 in, 2 out]
              }
              frame True {
                n257 = property on="Using Queue" class="Bool (strict)"("Val(Sgnl)"=FALSE ("Value (Signaling)")) -> ()  [unwired: 2 in, 2 out]
              }
            }
          }
        }
        n258 = call <vilib>:"Add State(s) to Queue__jki_lib_state_machine.vi"("State(s) in Front (\"\")"=w540, "State(s) in (\"\")"=w543) -> ("States Out"=w542:string)  [unwired: 13 in]
      }
      frame "-------Preset Execution----------" {
        # "Template Separator\n(You can make a copy of, or modify, this frame)"
        n259 = call <vilib>:"Add State(s) to Queue__jki_lib_state_machine.vi"("State(s) in (\"\")"=w570) -> ("States Out"=w569:string)  [unwired: 14 in]
      }
      frame "MC Control Update" {
        # "Template Separator\n(You can make a copy of, or modify, this frame)"
        n260 = disable-structure shown="Disabled" {
          disable-tunnel: w572 -> [w583 w584]
          disable-tunnel: [w576 w584] -> w571
          frame Disabled {
            n261 = Bundle By Name(cluster=w583, "Preset Manager Cluster.My IP"="My IP", "Preset Manager Cluster.Mcast address"="Mcast address", "Preset Manager Cluster.MCast Remote"="MCast Remote", "Preset Manager Cluster.UDP timeout ms"="UDP timeout ms", "Preset Manager Cluster.MC Multicast"="MC Multicast", "Preset Manager Cluster.All Devices Core Info"="All Devices Core Info") -> (w576:T6)
          }
          frame Enabled {
          }
        }
        n262 = call <vilib>:"Add State(s) to Queue__jki_lib_state_machine.vi"("State(s) in (\"\")"=w575) -> ("States Out"=w574:string)  [unwired: 14 in]
      }
      frame "General wait" {
        # "Template Separator\n(You can make a copy of, or modify, this frame)"
        n263 = call "get arguments of jki state.vi"("jki arguments"=w585) -> ("Arg 1"=w587:string)  [unwired: 1 in, 2 out]
        n264 = Decimal String To Number(string=w587) -> (number=w586:i32)  [unwired: 2 in, 1 out]
        n265 = Wait (ms)(milliseconds to wait=w586) -> ()  [unwired: 1 out]
        n266 = call <vilib>:"Add State(s) to Queue__jki_lib_state_machine.vi"("State(s) in (\"\")"=w591) -> ("States Out"=w590:string)  [unwired: 14 in]
      }
      frame "Poll Devices" {
        # "rem virt devs"
        # "Template Separator\n(You can make a copy of, or modify, this frame)"
        n267 = Unbundle By Name(w610) -> ("Preset Manager Cluster"=w609:T9)
        n268 = Unbundle By Name(w609) -> ("PresetName"=w596:string, "Current Preset Devices"=w605:string[], "All Devices Core Info"=w608:string[][], "Filtered Devices List"=w607:string[], "Virtual Devices List"=w606:string[], "DevStatusQueue"=w600:refnum<queue>)
        n269 = Preview Queue Element(queue=w600, timeout in ms (-1)=200) -> (element=w599:string[][], error out=→"error out":errorcluster)  [unwired: 1 in, 2 out]
        n270 = call "search string array for elements in 2nd string array.vi"("search for"=w606, "search in"=w607) -> ("Indices of Elements"=w611:i32[])  [unwired: 9 in]
        n271 = call-poly <userlib>:"Delete Elements from Array__ogtk.vi"("indices"=w611, "array"=w607) -> ("array w/ subset deleted"=w602:string[])  [unwired: 8 in, 1 out]
        n272 = call "get info from core device data.vi"("devices to get data from"=w602, "All Devices Core Info"=w608) -> ("IP Addresses"=w603:string[])  [unwired: 2 in, 1 out]
        n273 = Empty Array?(array=w603) -> (empty?=w604:bool)
        n274 = flat-sequence {
          tunnel: w605 -> [w621]
          tunnel: w604 -> [w620]
          tunnel: w603 -> [w619]
          tunnel: w602 -> [w618]
          tunnel: w599 -> [w617]
          tunnel: w596 -> [w615]
          tunnel: [w615] -> w593
          tunnel: [w616] -> w594
          tunnel: [w643] -> w597
          tunnel: w594 -> [w643]
          tunnel: w593 -> [w637]
          tunnel: [w636] -> w592
          frame #0 {
            n275 = case shown="False" w620 {
              tunnel: w615 -> [w628 _]
              tunnel: w621 -> [w627 _]
              tunnel: w619 -> [w626 _]
              tunnel: w618 -> [w625 _]
              tunnel: w617 -> [w623 _]
              tunnel: [w622 FALSE ("Active Preset Achieved")] -> w616
              frame False {
                # "Determine which devices are ON/OFF"
                n276 = call "get device status from tcp data array.vi"("TCP Device status data"=w623, "Current Preset Devices"=w627, "IP Addresses in"=w626, "Filtered Device List"=w625, "Requested Preset"=w628) -> ("Device Errors"=→"Device Errors":string[][], "Active boolean array"=→"Active Device array":bool[], "preset diagnostics"=w629:T13, "Active IP Addresses"=→"Active Dev/IP":string[], "Devices Not alive"=→"Devices not started":string[])  [unwired: 3 in, 3 out]
                n277 = Unbundle By Name(w629) -> ("Active Preset Achieved"=w622:bool)
                n278 = Select(t=w628, s=w622, f="Undefined") -> (s? t:f=→"Active Preset":string)
              }
              frame True {
              }
            }
          }
          frame #1 {
            n279 = property on="Active Preset" class="Str"() -> ("Value"=w639:string)  [unwired: 2 in, 2 out]
            n280 = property on="Poll Count" class="DigNum (strict)"() -> ("Value"=w641:i32)  [unwired: 2 in, 2 out]
            n281 = Not Equal?(x=w637, y=w639) -> (x != y?=w640:bool)
            n282 = Less?(x=w641, y=15) -> (x < y?=w642:bool)
            n283 = And(x=w640, y=w642) -> (x .and. y?=w636:bool)
          }
        }
        n284 = case shown="False" w592 {
          tunnel: w597 -> [w645 _]
          tunnel: [w644 "General Wait>>3000\nPoll Devices"] -> w595
          frame False {
            n285 = case shown="True" w645 {
              tunnel: ["" w651] -> w644
              frame False {
                n286 = property on="Preset Execution Indicator" class="Bool (strict)"("Blinking"=FALSE, "Caption.Text"=" Preset Failed" ("Boolean Text.Text"), "Value"=FALSE ("Blinking"), "Colors [4]"=cluster{u32, u32}[] [{16711680, 0}]) -> ()  [unwired: 2 in, 2 out]
              }
              frame True {
                n287 = property on="Using Queue" class="Bool (strict)"() -> ("Value"=w652:bool)  [unwired: 2 in, 2 out]
                n288 = property on="Preset Execution Indicator" class="Bool (strict)"("Blinking"=FALSE, "Caption.Text"=" Preset Executed" ("Boolean Text.Text"), "Value"=TRUE ("Blinking"), "Colors [4]"=cluster{u32, u32}[] [{318464, 0}]) -> ()  [unwired: 2 in, 2 out]
                n289 = case shown="True" w652 {
                  tunnel: ["" "Preset Queue Loading"] -> w651
                  frame False {
                  }
                  frame True {
                    n290 = property on="Queue Element" class="DigNum (strict)"() -> ("Value"=w660:i32)  [unwired: 2 in, 2 out]
                    n291 = Increment(x=w660) -> (x+1=w659:i32)
                    n292 = property on="Queue Element" class="DigNum (strict)"("Value"=w659) -> ()  [unwired: 2 in, 2 out]
                  }
                }
              }
            }
          }
          frame True {
            n293 = property on="Poll Count" class="DigNum (strict)"() -> ("Value"=w663:i32)  [unwired: 2 in, 2 out]
            n294 = Increment(x=w663) -> (x+1=w662:i32)
            n295 = property on="Poll Count" class="DigNum (strict)"("Value"=w662) -> ()  [unwired: 2 in, 2 out]
          }
        }
        n296 = call <vilib>:"Add State(s) to Queue__jki_lib_state_machine.vi"("State(s) in Front (\"\")"=w595, "State(s) in (\"\")"=w614) -> ("States Out"=w613:string)  [unwired: 13 in]
      }
      frame "Send Preset Command" {
        # "This State builds the Multicast Preset Command to all Devices"
        # "Template Separator\n(You can make a copy of, or modify, this frame)"
        n297 = Unbundle By Name(w670) -> ("Preset Manager Cluster.My IP"=w669:string, "Preset Manager Cluster.PresetName"=w665:string)
        n298 = call "preset SQL Queries.vi"("Expt name / MCIP/ Variable/Preset Name"=w665, "Preset Query"=Preset_Query_Enum."GetPresetDeviceNames") -> ("1st column 1st data"=w667:string[])  [unwired: 7 in, 2 out]
        n299 = Concatenate Strings("preset>>" ("string"), w665, ">>" ("string"), w669) -> (w668:string)
        n300 = Bundle By Name(cluster=w670, "Preset Manager Cluster.PresetName"=w665, "Preset Manager Cluster.Mcast command"=w668, "Preset Manager Cluster.Current Preset Devices"=w667) -> (w671:T6)
        n301 = property on="Poll Count" class="DigNum (strict)"("Value"=0) -> ()  [unwired: 2 in, 2 out]
        n302 = call <vilib>:"Add State(s) to Queue__jki_lib_state_machine.vi"("State(s) in (\"\")"=w677, "State(s) at Back (\"\")"="Send Multicast>>Empty\nGeneral wait>>10\nSend Multicast>>Empty\nGeneral wait>>40\nSend Multicast\nGeneral wait>>3000\nPoll Devices" ("Remaining States")) -> ("States Out"=w676:string)  [unwired: 13 in]
      }
      frame "Send Multicast" {
        # "Template Separator\n(You can make a copy of, or modify, this frame)"
        n303 = Unbundle By Name(w680) -> ("Preset Manager Cluster.MCast Remote"=w686:u16, "Preset Manager Cluster.Mcast address"=w685:string, "Preset Manager Cluster.UDP timeout ms"=w683:i32, "Preset Manager Cluster.Mcast command"=w682:string, "Preset Manager Cluster.MC Multicast"=w681:refnum<k16>)
        n304 = String To IP(1:w685) -> (0:w684:u32)
        n305 = UDP Write(address=w684, port or service name=w686, connection ID=w681, data in=w682, 9:w683) -> (3:w678:refnum<k16>)  [unwired: 1 in, 1 out]
        n306 = Bundle By Name(cluster=w680, "Preset Manager Cluster.MC Multicast"=w678) -> (w679:T6)
        n307 = call <vilib>:"Add State(s) to Queue__jki_lib_state_machine.vi"("State(s) in (\"\")"=w689) -> ("States Out"=w688:string)  [unwired: 14 in]
      }
      frame "-------------Diagnostics-----------" {
        # "Template Separator\n(You can make a copy of, or modify, this frame)"
        n308 = call <vilib>:"Add State(s) to Queue__jki_lib_state_machine.vi"("State(s) in (\"\")"=w693) -> ("States Out"=w692:string)  [unwired: 14 in]
      }
      frame "Execute Device Check" {
        # "Template Separator\n(You can make a copy of, or modify, this frame)"
        n309 = disable-structure shown="Enabled" {
          disable-tunnel: w695 -> [w701 _]
          disable-tunnel: [w700 _] -> w694
          frame Enabled {
            n310 = property on="Expt Devices Not On" class="LstBox (strict)"() -> ("Item Names"=w702:string[])  [unwired: 2 in, 2 out]
            n311 = property on="Preset Devices Not in Experiment" class="LstBox (strict)"() -> ("Item Names"=w703:string[])  [unwired: 2 in, 2 out]
            n312 = call-poly <userlib>:"Empty Array__ogtk.vi"("Array"=w702) -> ("Empty Array?"=w705:bool)  [unwired: 8 in]
            n313 = call-poly <userlib>:"Empty Array__ogtk.vi"("Array"=w703) -> ("Empty Array?"=w706:bool)  [unwired: 8 in]
            n314 = And(x=w706, y=w705) -> (x .and. y?=w704:bool)
            n315 = case shown="False" w704 {
              tunnel: [w707 w719] -> w700
              tunnel: w701 -> [w708 w719]
              frame False {
                n316 = Two Button Dialog(message="There are either some presets that are not in the \\n\nexperiment or some devices are not on. Please \\n\nif that would impact the preset excution. ", 1:"Stop Execution" ("F button name (\"Cancel\")"), 2:"Continue Execution" ("T button name (\"OK\")")) -> (T button?=w712:bool)
                n317 = case shown="False" w712 {
                  tunnel: ["" ("State(s) in Front (\"\")") w718] -> w707
                  tunnel: w708 -> [_ w718]
                  frame False {
                    w713 = FALSE
                    n318 = control-ref of="Preset Execution Indicator"() -> (w716:refnum<vi>)
                    n319 = property on="Queue Size" class="DigNum (strict)"("Visible"=w713) -> ()  [unwired: 2 in, 2 out]
                    n320 = property on="Current Preset Queue Element" class="Str"("Visible"=w713) -> ()  [unwired: 2 in, 2 out]
                    n321 = property on="Queue Progress Bar" class="Slide (strict)"("Visible"=w713) -> ()  [unwired: 2 in, 2 out]
                    n322 = property on="Property Node" class="Bool (strict)"(reference=w716, "Blinking"=FALSE, "Caption.Text"="" ("Boolean Text.Text")) -> ()  [unwired: 1 in, 2 out]
                  }
                  frame True {
                  }
                }
              }
              frame True {
              }
            }
          }
          frame Disabled {
          }
        }
        n323 = call <vilib>:"Add State(s) to Queue__jki_lib_state_machine.vi"("State(s) in Front (\"\")"=w694, "State(s) in (\"\")"=w699) -> ("States Out"=w698:string)  [unwired: 13 in]
      }
      frame "Expt Device Check" {
        # "Template Separator\n(You can make a copy of, or modify, this frame)"
        n324 = flat-sequence {
          tunnel: w721 -> [w739]
          tunnel: w720 -> [w734]
          frame #0 {
            n325 = call <vilib>:"Set Busy.vi"("disable click? (T)"=TRUE, "cursor ID"=refnum<k1> refnum) -> ()  [unwired: 8 in, 2 out]
          }
          frame #1 {
            n326 = Unbundle By Name(w739) -> ("Preset Manager Cluster.Experiment Name"=w730:string, "Preset Manager Cluster.PresetName"=w738:string, "Preset Manager Cluster.All Devices Core Info"=w729:string[][], "Preset Manager Cluster.DevStatusQueue"=w728:refnum<queue>)
            n327 = Equal?(x=w734, y="Preset Only") -> (x = y?=w733:bool)
            n328 = case shown="True" w733 {
              tunnel: [enum16{"Preset Queue", "Preset Only"}."Preset Queue" ("Input Type") enum16{"Preset Queue", "Preset Only"}."Preset Only" ("Input Type")] -> w732
              frame False {
              }
              frame True {
              }
            }
            n329 = property on="Queue Table" class="Tbl (strict)"() -> ("Value"=w731:string[][])  [unwired: 2 in, 2 out]
            n330 = call "Preset Expt Device Comparison.vi"("Input Type"=w732, "Preset Name"=w738, "Preset Array"=w731, "Expt name"=w730) -> ("Devices Not in Experiment"=w736:string[], "Devices accounted for?"=w737:bool)  [unwired: 6 in]
            n331 = property on="Preset Devices Not in Experiment" class="LstBox (strict)"("Item Names"=w736) -> ()  [unwired: 2 in, 2 out]
            n332 = call "Devices Not On.vi"("All Devices Core Info"=w729, "Experiment"=w730, "queue"=w728) -> ("Devices Not alive"=w727:string[])  [unwired: 8 in]
            n333 = property on="Expt Devices Not On" class="LstBox (strict)"("Item Names"=w727) -> ()  [unwired: 2 in, 2 out]
            n334 = case shown="True" w737 {
              frame False {
                n335 = property on="Preset Execution Indicator" class="Bool (strict)"("Blinking"=FALSE, "Caption.Text"="Devices Not \nin Experiment" ("Boolean Text.Text"), "Value"=FALSE ("Blinking"), "Colors [4]"=cluster{u32, u32}[] [{16711680, 0}]) -> ()  [unwired: 2 in, 2 out]
              }
              frame True {
                n336 = property on="Preset Execution Indicator" class="Bool (strict)"("Blinking"=FALSE, "Caption.Text"="" ("Boolean Text.Text"), "Value"=FALSE ("Blinking"), "Colors [4]"=cluster{u32, u32}[] [{32639, 0}]) -> ()  [unwired: 2 in, 2 out]
              }
            }
          }
          frame #2 {
            n337 = call <vilib>:"Unset Busy.vi"() -> ()  [unwired: 11 in, 1 out]
          }
        }
        n338 = call <vilib>:"Add State(s) to Queue__jki_lib_state_machine.vi"("State(s) in (\"\")"=w724) -> ("States Out"=w723:string)  [unwired: 14 in]
      }
      frame "Check Expt Device On" {
        # "Template Separator\n(You can make a copy of, or modify, this frame)"
        n339 = Unbundle By Name(w754) -> ("Preset Manager Cluster.Experiment Name"=w753:string, "Preset Manager Cluster.All Devices Core Info"=w752:string[][], "Preset Manager Cluster.DevStatusQueue"=w751:refnum<queue>)  [unwired: 1 out]
        n340 = call "Devices Not On.vi"("All Devices Core Info"=w752, "Experiment"=w753, "queue"=w751) -> ("Devices Not alive"=w750:string[])  [unwired: 8 in]
        n341 = property on="Expt Devices Not On" class="LstBox (strict)"("Item Names"=w750) -> ()  [unwired: 2 in, 2 out]
        n342 = call <vilib>:"Add State(s) to Queue__jki_lib_state_machine.vi"("State(s) in (\"\")"=w757) -> ("States Out"=w756:string)  [unwired: 14 in]
      }
    }
  }
